vi "Navigation_start_cases.vi"() -> ()   [LabVIEW 2015]
uses:
  <vilib>/myRIO/Instrument Drivers/Onboard IO/PWM/typedefs/PWM Reference.ctl
  <vilib>/myRIO/Common/Instrument Driver Framework/Utilities/typedefs/myRIO Generic Hardware Reference.ctl
  <vilib>/myRIO/Common/Instrument Driver Framework/Utilities/typedefs/Hardware Version Enum.ctl
  <vilib>/myRIO/Common/Instrument Driver Framework/Utilities/typedefs/myRIO v1.0 Reference.ctl
  <vilib>/myRIO/Common/Instrument Driver Framework/Utilities/typedefs/Generic FPGA Reference.ctl
  <vilib>/myRIO/Common/Instrument Driver Framework/myRIO v1.0/PWM/typedefs/PWM Channels Enum.ctl
  <vilib>/myRIO/Instrument Drivers/Onboard IO/PWM/typedefs/PWM Configuration.ctl
  <vilib>/userdefined/High Color/nirio_resource_hc.ctl
  <vilib>/myRIO/Common/Instrument Driver Framework/myRIO v1.0/PWM/vis/myRIO v1.1 Open PWM.vi
  <vilib>/myRIO/Common/Instrument Driver Framework/Utilities/vis/Validate Channels.vi
  <vilib>/myRIO/Common/Instrument Driver Framework/myRIO v1.0/PWM/vis/myRIO v1.0 Reserve PWM.vi
  <vilib>/myRIO/Common/Instrument Driver Framework/myRIO v1.0/PWM/vis/myRIO v1.0 Build MUX Configuration PWM.vi
  <vilib>/myRIO/Common/Instrument Driver Framework/myRIO v1.0/Resource Manager/vis/myRIO v1.0 Reserve Channel List.vi
  <vilib>/myRIO/Common/Instrument Driver Framework/myRIO v1.0/Resource Manager/vis/myRIO v1.0 Create Configuration List.vi
  <vilib>/myRIO/Common/Instrument Driver Framework/myRIO v1.0/Resource Manager/vis/myRIO v1.0 Reserve Channel.vi
  <vilib>/myRIO/Common/Instrument Driver Framework/myRIO v1.0/Resource Manager/vis/myRIO v1.0 Unreserve Channel.vi
  <vilib>/myRIO/Common/Instrument Driver Framework/myRIO v1.0/Resource Manager/vis/myRIO v1.0 Build Mutex Name.vi
  <vilib>/FPGAPlugInAG/myRIO-1900/niLvFpga_Open_myRIO-1900.vi
  <vilib>/rvi/interface/common/dynamic/niFpgaDynamicAddResources.vi
  <vilib>/myRIO/Common/Instrument Driver Framework/Utilities/vis/FPGA Ref Manager.vi
  <vilib>/Utility/error.llb/Error Cluster From Error Code.vi
  <vilib>/myRIO/Common/Instrument Driver Framework/Utilities/vis/Ref Counter.vi
  <vilib>/rvi/errors/niLvFpgaAdjustHostInterfaceError.vi
  <vilib>/Utility/VariantDataType/GetNumericInfo.vi
  <vilib>/myRIO/Common/Instrument Driver Framework/myRIO v1.0/myRIO v1.1 Open.vi
  <vilib>/myRIO/Common/Instrument Driver Framework/Utilities/vis/IO Manager.vi
  <vilib>/myRIO/Common/Instrument Driver Framework/Utilities/vis/Configuration Manager.vi
  <vilib>/myRIO/Common/Instrument Driver Framework/myRIO v1.0/Resource Manager/vis/myRIO v1.0 Configure IO.vi
  <vilib>/myRIO/Common/Instrument Driver Framework/myRIO v1.0/myRIO v1.0 Close.vi
  <vilib>/myRIO/Common/Instrument Driver Framework/myRIO v1.0/PWM/vis/myRIO v1.0 Write PWM.vi
  <vilib>/addons/control/pid/pid.llb/PID (DBL).vi
  <vilib>/rvi/interface/nirviOpenFPGA/nirviOpenFPGA.xnode
  FPGA Bitfiles/NavigationProjec_FPGATarget2_FPGAMainNavigati_PWPHW8gwDxI.lvbitx
  <vilib>/rvi/interface/nirviReadWriteControl/nirviReadWriteControl.xnode
  <vilib>/myRIO/Instrument Drivers/Onboard IO/PWM/vis/myRIO PWM Open.xnode
  <vilib>/myRIO/Instrument Drivers/Onboard IO/PWM/PWM.lvlib
  <vilib>/myRIO/Instrument Drivers/Utilities/Utilities.lvlib
  NiFpgaLv.dll
  <vilib>/rvi/interface/Simulation/niFpgaSimulationCallBeginRW.vi
  <vilib>/addons/control/pid/NI_PID_pid.lvlib
panel:
  in  "t backward 6":u32=3000
  in  "Tab Control":enum32{"start a", "start b"}(tab)
  in  "?":T1(tab)=enum."back arc 4 4"
  in  "right 0":dbl=-0.05
  in  "left 0":dbl=-0.05
  in  "t backward 7":u32=3000
  in  "left 1":dbl=0.1
  in  "right 1":dbl=0.05
  in  "right 2":dbl=0.05
  in  "left 2":dbl=0.1
  in  "t backward":u32=3000
  in  "t forward":u32=750
  in  "t forward once":u32=3000
  in  "right once":dbl=0.05
  in  "left once":dbl=0.1
  in  "left 7":dbl=0.1
  in  "right 7":dbl=0.05
  in  "t forward 2":u32=750
  in  "left 6":dbl=0.1
  in  "right 6":dbl=0.05
  in  "t backward 2":u32=3000
  in  "left once 2":dbl=0.1
  in  "right once 2":dbl=0.05
  in  "t forward once 2":u32=3000
  in  "left 12":dbl=0.1
  in  "right 12":dbl=0.05
  in  "left 11":dbl=0.1
  in  "right 11":dbl=0.05
  in  "left 10":dbl=0.1
  in  "right 10":dbl=0.05
  in  "forward":u32=5000
  in  "timeforward":u32=750
  in  "timeback":u32=750
  in  "Tab Control 3":T2(tab)
  in  "left 15":dbl=-0.05
  in  "right 15":dbl=-0.05
  in  "t backward 8":u32=3000
  in  "left 5":dbl=0.1
  in  "right 5":dbl=0.05
  in  "left 4":dbl=0.1
  in  "right 4":dbl=0.05
  in  "left 3":dbl=0.1
  in  "right 3":dbl=0.05
  in  "forward 6":u32=750
  in  "backward 6":u32=750
  in  "onetime 6":u32=5000
  in  "t forward once 5":u32=3000
  in  "right once 5":dbl=0.05
  in  "left once 5":dbl=0.1
  in  "left 16":dbl=0.1
  in  "right 16":dbl=0.05
  in  "t backward 5":u32=3000
  in  "left 17":dbl=0.1
  in  "right 17":dbl=0.05
  in  "t forward 5":u32=750
  in  "start condition":dbl=4.0
  out "percent to goal":dbl
  out "x goal current":dbl=8.0
  out "big red button":i16
  out "y1ahead":dbl
  out "angle error":dbl
  out "y desired":dbl
  out "slope desired":dbl
  out "orientation theta desired":dbl
  out "current angle":dbl
  out "current y":dbl
  out "current x":dbl
  out "mining angle":dbl
  out "mining y":dbl
  out "mining x":dbl
  out "mining location":dbl=1.0
  out "distance to goal":dbl
  out "loc_y":dbl
  out "loc_x":dbl
  out "loc_theta":dbl
  in  "motor killswitch":bool=TRUE
  in  "set start position":bool
  in  "dumping complete":bool
  in  "digging complete?":bool
  in  "position good?":bool
  in  "state":dbl=5.0
  in  "x goal":dbl=8.0
  in  "Encoder Reset":bool
  out "scale":dbl=1.0
  out "reset x y 2":dbl
  out "stop motors":dbl
  out "encoder stop switch":dbl=1.0
  out "left wheels actual pwm":dbl
  out "right wheels actual pwm":dbl
  out "desired pwm right":dbl
  out "desired pwm left":dbl
  out "left setpoint":dbl
  out "right setpoint":dbl
  in  "PID Settings":enum32{"Right PID PWM", "Left PID PWM"}(tab)
  in  "output range right":cluster{"output high":dbl, "output low":dbl}={"output high"=0.13333, "output low"=-0.13333} {"output low" format="%.6f"; "output high" format="%.5f"}
  in  "PID gains right":T3={"proportional gain (Kc)"=0.002, "integral time (Ti, min)"=7e-07, "derivative time (Td, min)"=0.0} {"derivative time (Td, min)" format="%.8f"; "integral time (Ti, min)" format="%.8f"; "proportional gain (Kc)" format="%.8f"}
  out "dt out (s) right":dbl format="%.3f"
  out "PID feedback Right":dbl
  out "Elapsed Time (s) Right":dbl caption="Elapsed Time (s)"
  in  "pid reset right":bool
  in  "output range left":cluster{"output high":dbl, "output low":dbl}={"output high"=0.13333, "output low"=-0.13333} {"output low" format="%.6f"; "output high" format="%.5f"}
  in  "PID gains left":T3={"proportional gain (Kc)"=0.002, "integral time (Ti, min)"=7e-07, "derivative time (Td, min)"=0.0} {"derivative time (Td, min)" format="%.8f"; "integral time (Ti, min)" format="%.8f"; "proportional gain (Kc)" format="%.8f"}
  out "dt out (s) left":dbl format="%.3f"
  out "PID feedback Left":dbl
  out "Elapsed Time (s) Left":dbl caption="Elapsed Time (s)"
  in  "pid reset left":bool
  out "start angle":dbl=1.0
  out "start x":dbl=1.0
  out "start y":dbl
  in  "stuff that i dont want to mess with right now":T4(tab)
  out "RM Linear Velocity (rot/s)":dbl
  out "RR Rot Velocity (rot/s)":dbl
  out "LR Rot Velocity (rot/s)":dbl
  out "LM Rot Velocity (rot/s)":dbl
  out "LF Rot Velocity (rot/s)":dbl
  out "RF Linear Velocity (rot/s)":dbl
  out "Tick Count(mSec) 2":u32 caption="Tick Count(mSec)"
  out "y traveled 2":dbl
  out "x traveled 2":dbl
  out "y position 2":dbl
  out "x position 2":dbl
  out "y dot 2":dbl
  out "distance traveled 2":dbl
  out "psi dot 2":dbl
  out "x dot 2":dbl
  out ".not. x? 2":bool
  out ".not. x? 3":bool
  out "goal reached":bool=TRUE
  out "avg ENC.B":dbl
  out "avg ENC.A":dbl
  out "ENC.B_c.CNTR":i32
  out "ENC.B_b.CNTR":i32
  out "ENC.B_a.CNTR":i32
  out "ENC.A_c.CNTR":i32
  out "ENC.A_b.CNTR":i32
  out "ENC.A_a.CNTR":i32
  out "stage set point parameters":T5(tab)
  in  "x straight 1 end":dbl=2.0
  in  "ypstart straight 1":dbl
  in  "ystart":dbl=1.0
  in  "yend straight 1":dbl=2.0
  in  "ypend straight 1":dbl
  out "a":dbl
  out "b":dbl
  out "c":dbl
  out "d":dbl
  out "x turn end":dbl=7.0
  out "x straight 2 end":dbl=10.0
  in  "mining y 1":dbl=2.0
  in  "mining angle 1":dbl
  in  "mining x 1":dbl=-8.0
  in  "mining angle -1":dbl
  in  "mining y -1":dbl=4.0
  in  "mining x -1":dbl=-8.0
  out "left pwm":dbl(graph)
  out "right pwm":dbl(graph)
  out "SYS.SELECTA":u8 format="%08b"
  in  "R Min Linear Velocity (ft/s)":dbl=-2.0 format="%#_13g"
  in  "R Max Linear Velocity (ft/s)":dbl=2.0 format="%#_13g"
  in  "L Min Linear Velocity (ft/s)":dbl=-2.0 format="%#_13g"
  in  "L Max Linear Velocity (ft/s)":dbl=2.0 format="%#_13g"
  out "Current Rot Velocity (rot/s)":T6(graph)
  # "Position Information"
  # "straight arc back straight arc arc"
  # "same as the start a arc arc"
  # "move cases along"
  # "end state 0\ngo to state 1"
  # "end state 1\ngo to state 2"
  # "end state 2\ngo to state 3"
  # "end state 3\ngo to state 4"
  # "end state 4\ngo to state 0"
  # "same thing, redundant \nbut can be changed to \nsomething useful later"
  # "this must be true to \ninitialize the routine"
  # "go through the 3\n movement cases"
  # "go through the 3\n movement cases"
  # "Stop Flags \n1=go \n0=stop"
  # "PWM Setpoint"
  # "Initial condtions"
  # "Encoder Values"
  # "Motor Control Parameters"
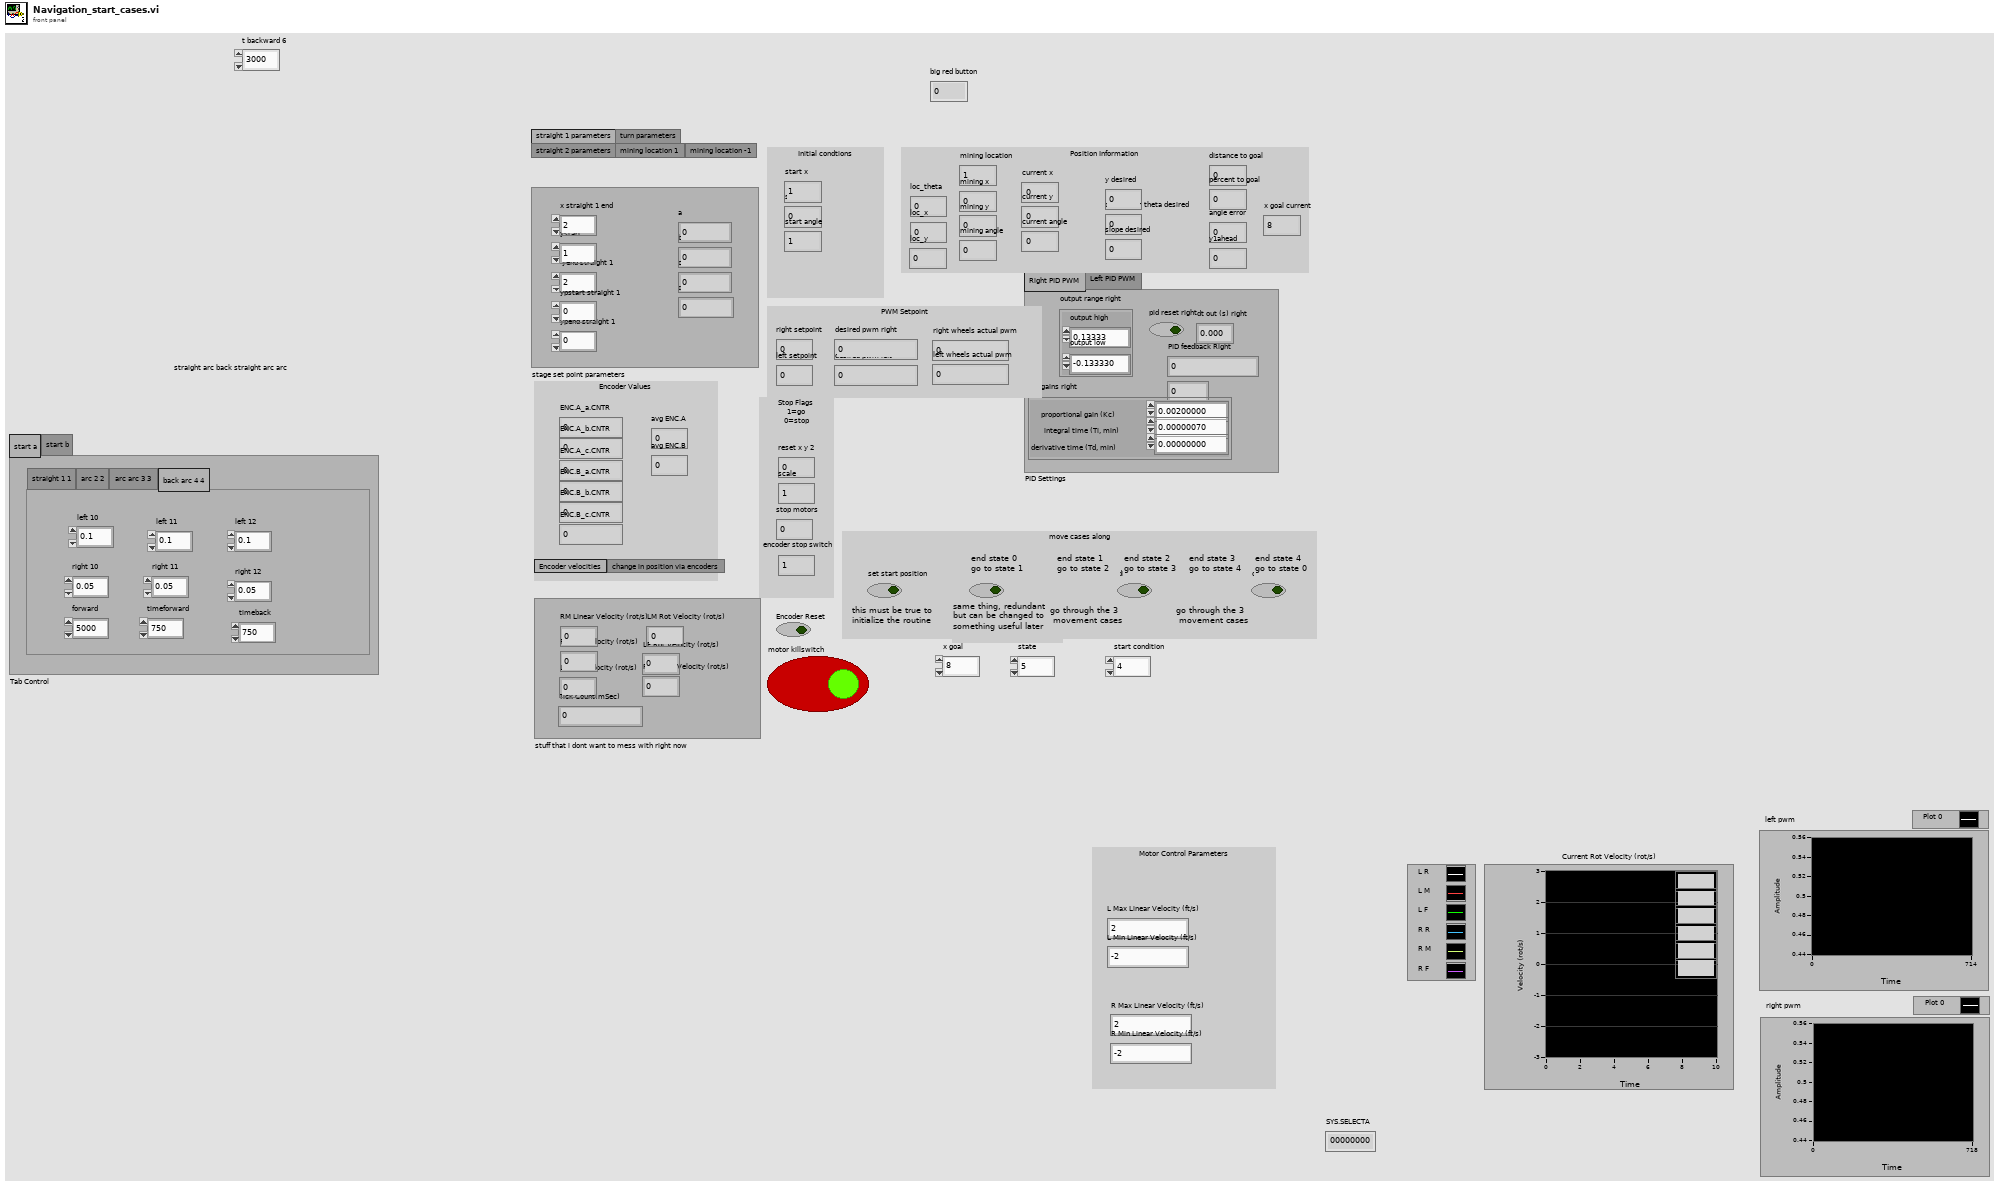
[diagram p1: front panel]
types:
  T1 = enum32{"straight 1 1", "arc 2 2", "arc arc 3 3 ", "back arc 4 4"}
  T2 = enum32{"straight 1 5", "arc 2 6", "arc arc 3", "back arc 4 7"}
  T3 = cluster{"proportional gain (Kc)":dbl, "integral time (Ti, min)":dbl, "derivative time (Td, min)":dbl}
  T4 = enum32{"Encoder velocities", "change in position via encoders"}
  T5 = enum32{"straight 1 parameters", "turn parameters", "straight 2 parameters", "mining location 1", "mining location -1"}
  T6 = cluster{"Rotational Velocity (RPS)":dbl, "Rotational Velocity (RPS)":dbl, "Rotational Velocity (RPS)":dbl, "Rotational Velocity (RPS)":dbl, "Rotational Velocity (RPS)":dbl, "Rotational Velocity (RPS)":dbl}
  T7 = typedef "nirio_resource_hc.ctl" = tag
  T8 = typedef "Hardware Version Enum.ctl" = enum16{"Unknown", "myRIO-1900", "myRIO-1950", "roboRIO"}
  T9 = typedef "PWM.lvlib/PWM Reference.ctl" = cluster{"myRIO Reference":T10, "PWM Channels Enum":T13, "PWM Configuration":T14}
  T10 = typedef "myRIO Generic Hardware Reference.ctl" = cluster{"myRIO Model":T8, "myRIO Hardware Reference":T11}
  T11 = typedef "myRIO v1.0 Reference.ctl" = cluster{"Generic FPGA Reference":T12, "Allow multiple opens":bool}
  T12 = typedef "Generic FPGA Reference.ctl" = refnum<k20>
  T13 = typedef "PWM Channels Enum.ctl" = enum16{"Not Connected", "C/PWM0", "C/PWM1", "A/PWM0", "A/PWM1", "A/PWM2", "B/PWM0", "B/PWM1", "B/PWM2", "PWM/PWM0", "PWM/PWM1", "PWM/PWM2", "PWM/PWM3", "PWM/PWM4", "PWM/PWM5", "PWM/PWM6", "PWM/PWM7", "PWM/PWM8", "PWM/PWM9"}
  T14 = typedef "PWM.lvlib/PWM Configuration.ctl" = cluster{"Frequency":dbl, "Duty Cycle":dbl}
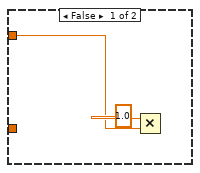
[diagram p3: hidden frame]
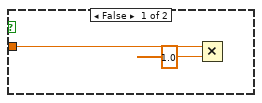
[diagram p4: hidden frame]
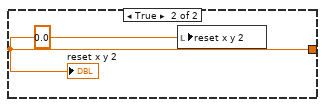
[diagram p5: hidden frame]
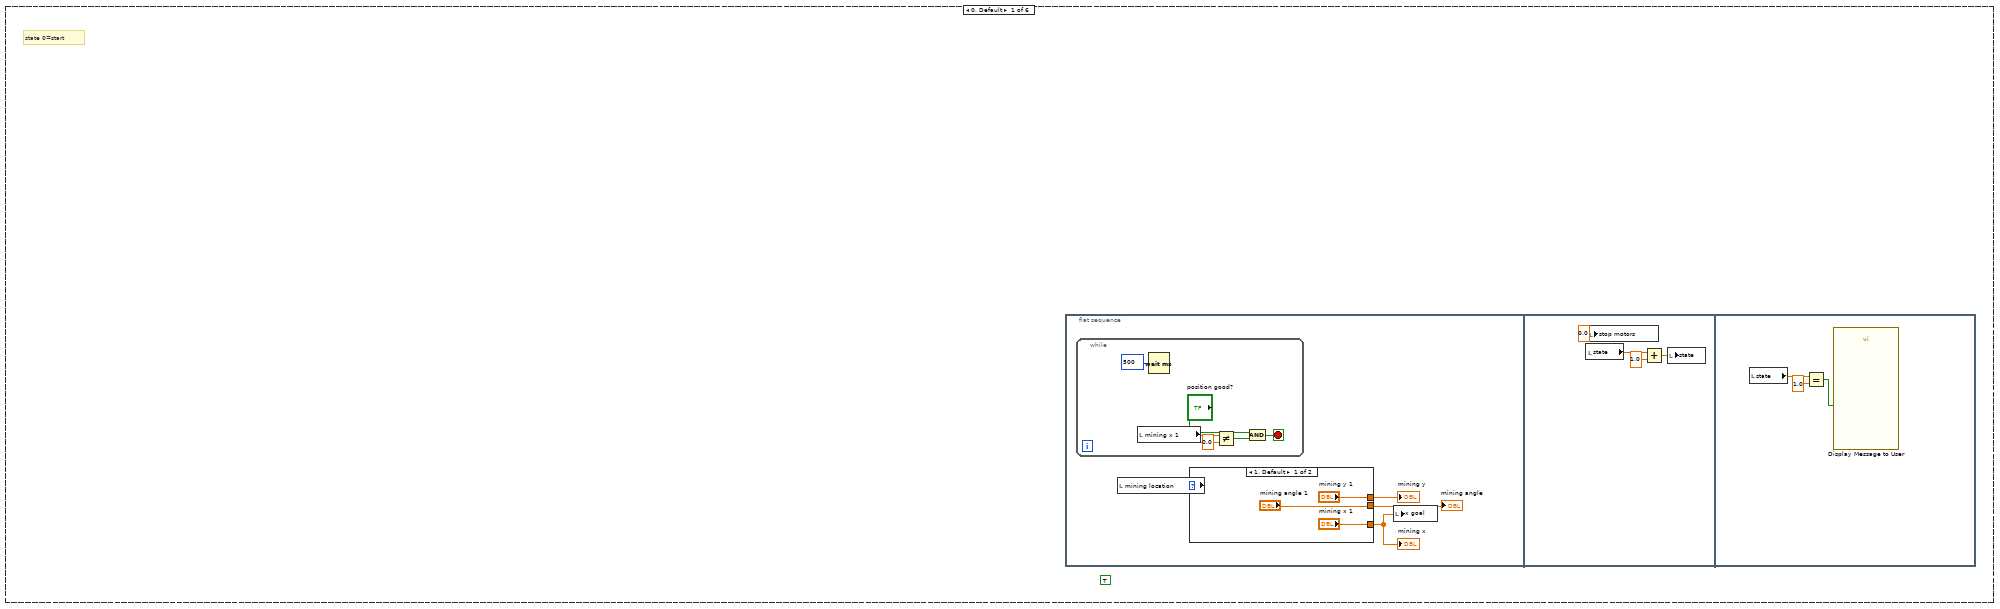
[diagram p6: hidden frame]
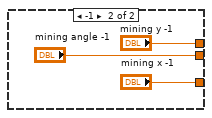
[diagram p7: hidden frame]
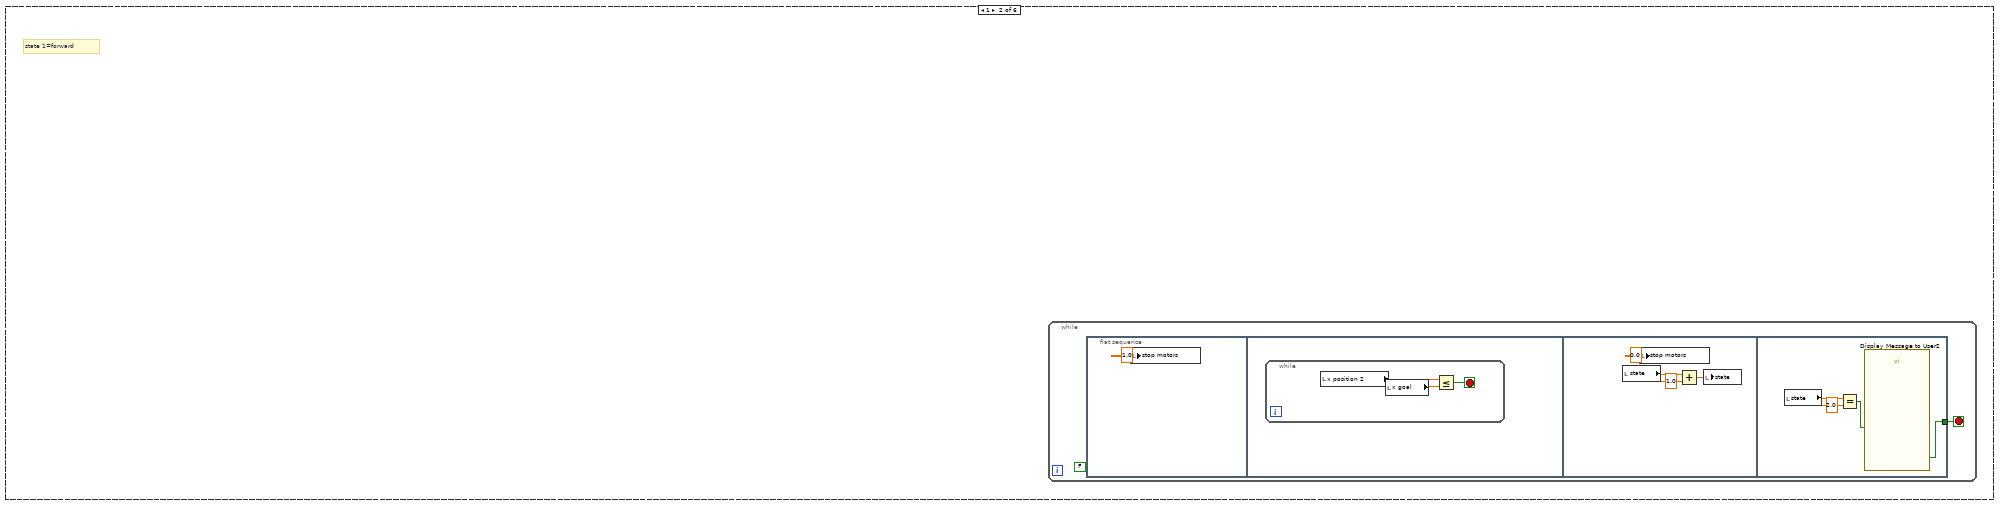
[diagram p8: hidden frame]
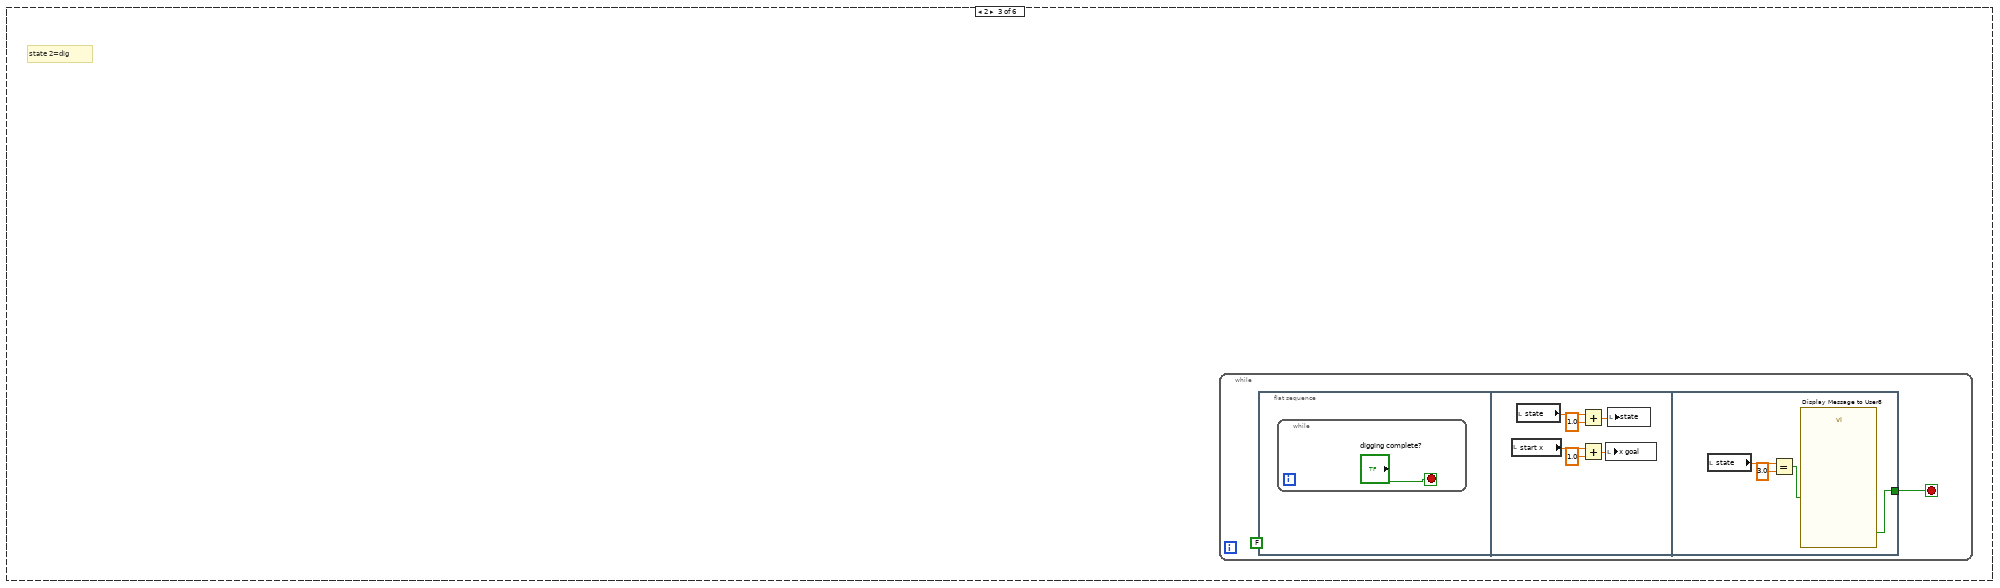
[diagram p9: hidden frame]
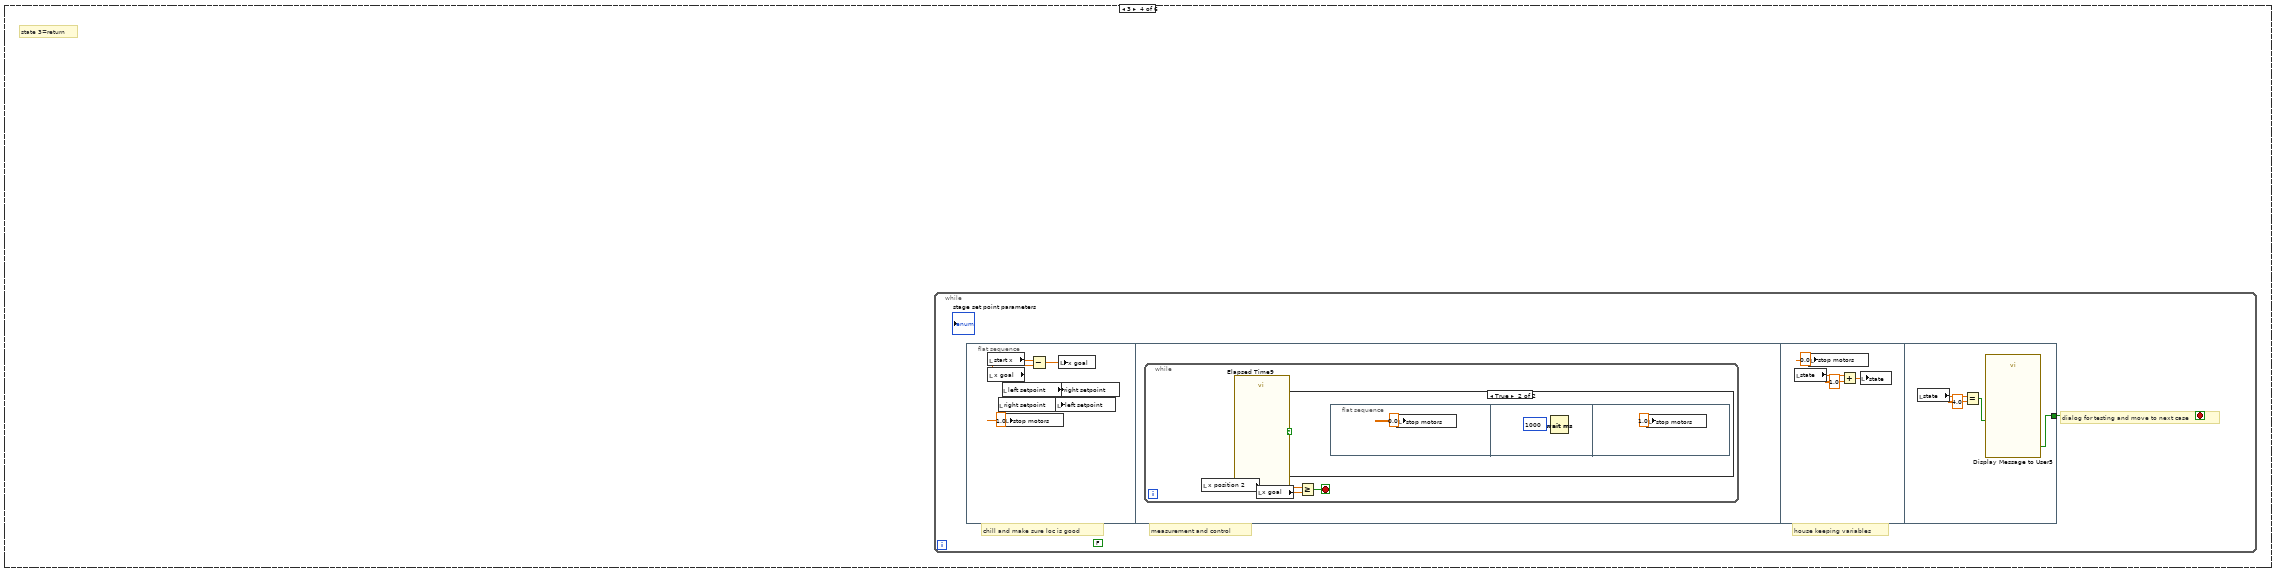
[diagram p10: hidden frame]
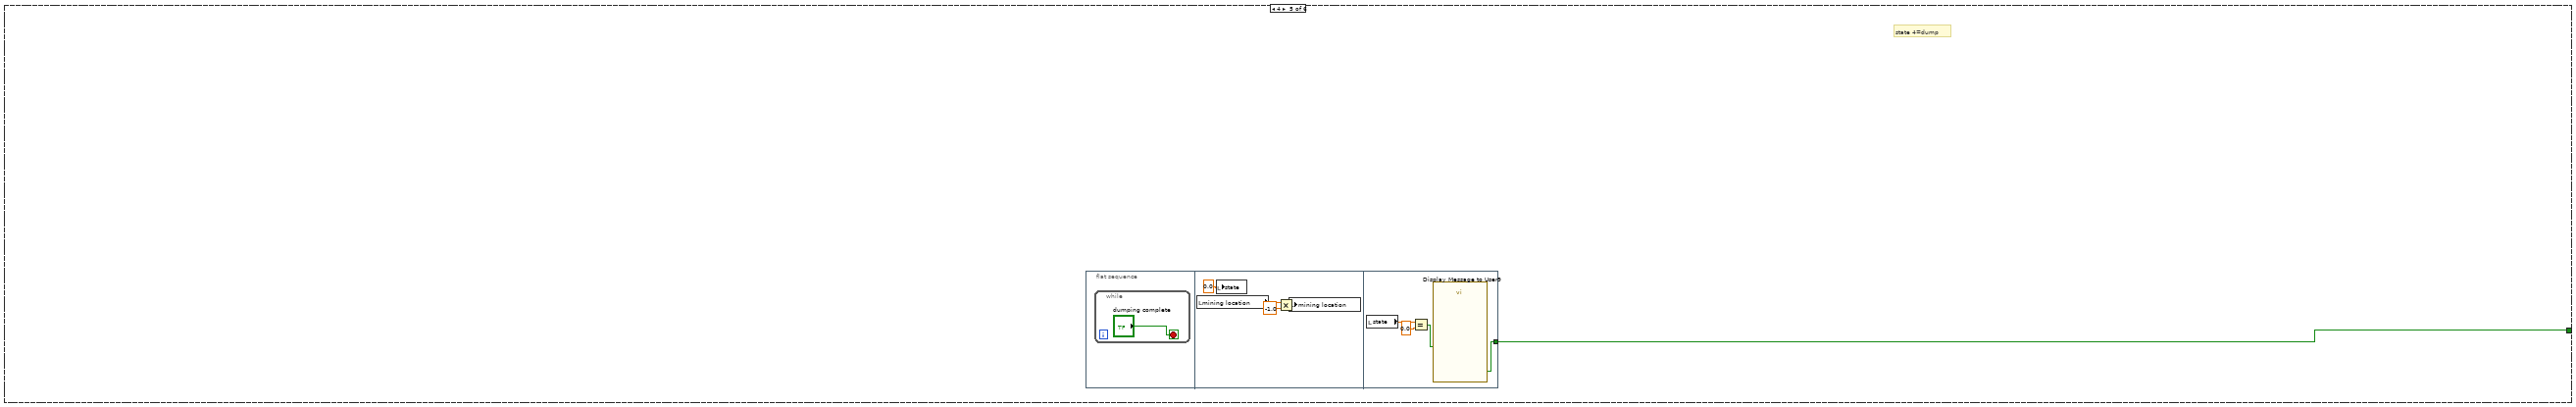
[diagram p12: hidden frame]
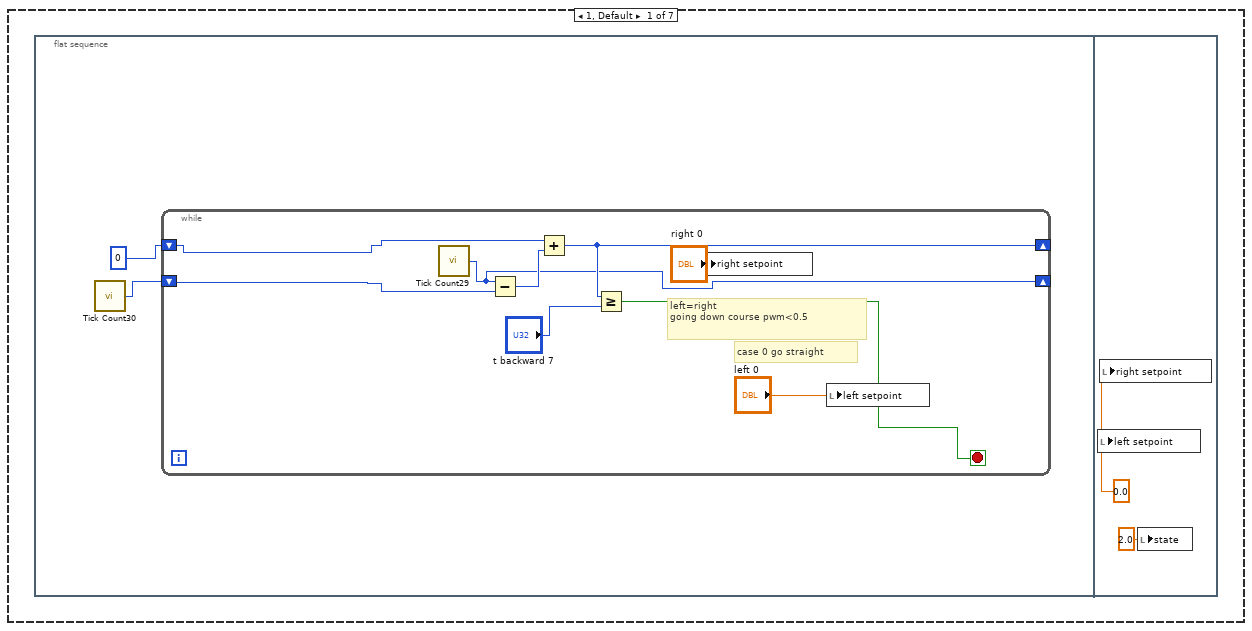
[diagram p13: hidden frame]
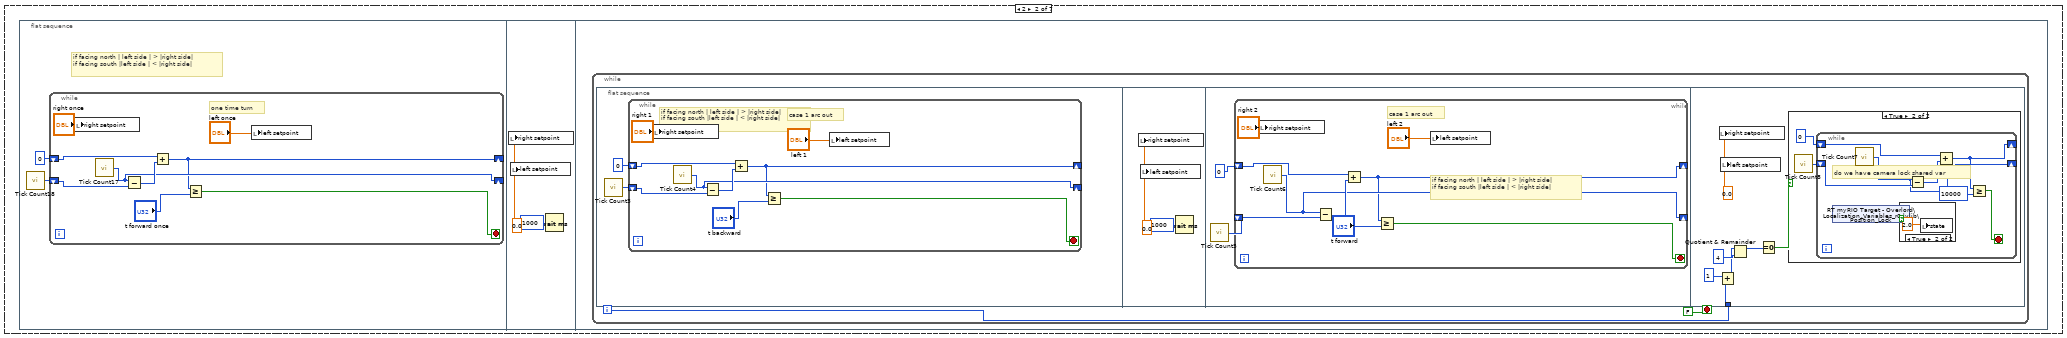
[diagram p14: hidden frame]
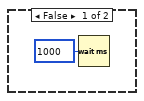
[diagram p15: hidden frame]
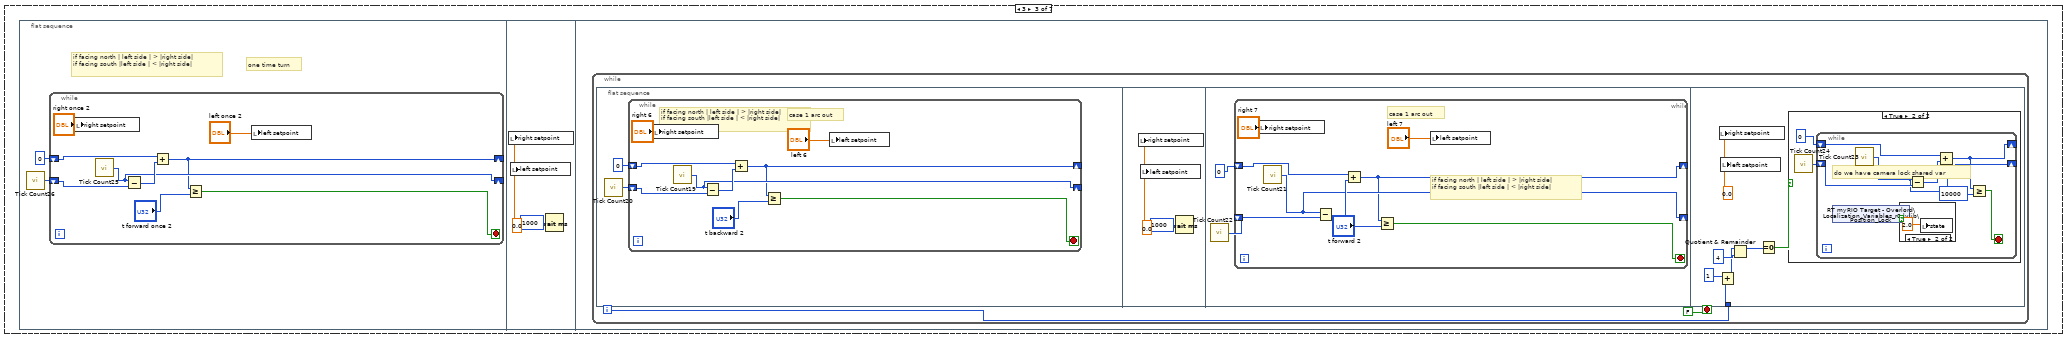
[diagram p17: hidden frame]
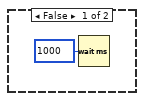
[diagram p18: hidden frame]
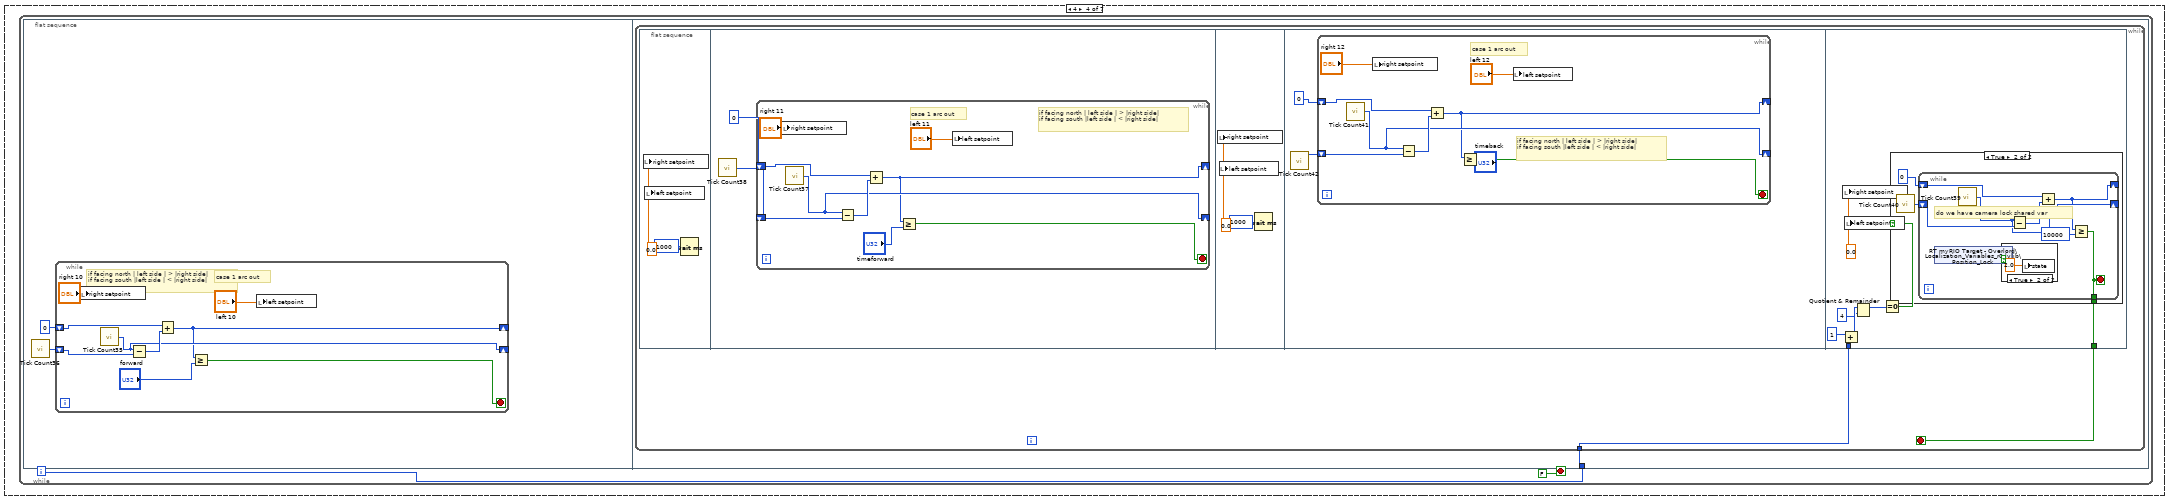
[diagram p20: hidden frame]
diagram:
  n1 = flat-sequence {
    tunnel: [w33] -> w30
    tunnel: [w33] -> w29
    tunnel: [w46] -> w28
    tunnel: [w61] -> w26
    tunnel: [w57] -> w24
    tunnel: [w56] -> w22
    tunnel: [w55] -> w20
    tunnel: [w54] -> w18
    tunnel: [w53] -> w16
    tunnel: ["L Max Linear Velocity (ft/s)"] -> w14
    tunnel: ["L Min Linear Velocity (ft/s)"] -> w12
    tunnel: ["R Max Linear Velocity (ft/s)"] -> w10
    tunnel: ["R Min Linear Velocity (ft/s)"] -> w8
    tunnel: [w48] -> w6
    tunnel: w30 -> [w47]
    tunnel: [w47] -> w4
    tunnel: w29 -> [w48]
    tunnel: [w46] -> w2
    tunnel: w28 -> [w187]
    tunnel: [w187] -> w27
    tunnel: w26 -> [w186]
    tunnel: [w186] -> w25
    tunnel: w24 -> [w185]
    tunnel: [w185] -> w23
    tunnel: w22 -> [w184]
    tunnel: [w184] -> w21
    tunnel: w20 -> [w183]
    tunnel: [w183] -> w19
    tunnel: w18 -> [w182]
    tunnel: [w182] -> w17
    tunnel: w16 -> [w181]
    tunnel: [w181] -> w15
    tunnel: w14 -> [w180]
    tunnel: [w180] -> w13
    tunnel: w12 -> [w179]
    tunnel: [w179] -> w11
    tunnel: w10 -> [w178]
    tunnel: [w178] -> w9
    tunnel: w8 -> [w177]
    tunnel: [w177] -> w7
    tunnel: w6 -> [w176]
    tunnel: [w176] -> w5
    tunnel: w4 -> [w175]
    tunnel: [w175] -> w3
    tunnel: w2 -> [w174]
    tunnel: [w174] -> w1
    tunnel: w27 -> [_]
    tunnel: w25 -> [w198]
    tunnel: w23 -> [w204]
    tunnel: w21 -> [w201]
    tunnel: w19 -> [w200]
    tunnel: w17 -> [w199]
    tunnel: w15 -> [w203]
    tunnel: w13 -> [_]
    tunnel: w11 -> [_]
    tunnel: w9 -> [_]
    tunnel: w7 -> [_]
    tunnel: w5 -> [w206]
    tunnel: w3 -> [w205]
    tunnel: w1 -> [w202]
    frame #0 {
      n2 = xnode "Open FPGA VI Reference"("resource name"=tag "RIO0") -> ("FPGA VI Reference Out"=w32:refnum<k20>)  [unwired: 1 in, 1 out]
      n3 = call <vilib>:"Set Custom Bitfile.vi"("Custom FPGA Reference In"=w32) -> ("Custom FPGA Reference Out"=w34:refnum<k20>)  [unwired: 9 in, 1 out]
      n4 = flat-sequence {
        tunnel: w34 -> [w39]
        tunnel: [w37] -> w36
        tunnel: w36 -> [w41]
        tunnel: [w41] -> w35
        tunnel: w35 -> [w44]
        tunnel: [w43] -> w33
        frame #0 {
          w38 = u8 32 ("SYS.SELECTA")
          w40 = u8 3 ("ENC.B_c.CNFG")
          n5 = xnode "Read/Write Control"("FPGA VI Reference In"=w39, "ENC.A_a.CNFG"=w40, "ENC.A_b.CNFG"=w40, "ENC.A_c.CNFG"=w40, "ENC.B_a.CNFG"=w40, "ENC.B_b.CNFG"=w40, "ENC.B_c.CNFG"=w40, "SYS.SELECTA"=w38, "SYS.SELECTB"=w38) -> ("FPGA VI Reference Out"=w37:refnum<k20>)  [unwired: 1 in, 1 out]
        }
        frame #1 {
          n6 = Wait (ms)(milliseconds to wait=u32 10) -> ()  [unwired: 1 out]
        }
        frame #2 {
          w45 = u8 1 ("ENC.B_c.CNFG")
          n7 = xnode "Read/Write Control"("FPGA VI Reference In"=w44, "ENC.A_a.CNFG"=w45, "ENC.A_b.CNFG"=w45, "ENC.A_c.CNFG"=w45, "ENC.B_a.CNFG"=w45, "ENC.B_b.CNFG"=w45, "ENC.B_c.CNFG"=w45) -> ("FPGA VI Reference Out"=w43:refnum<k20>)  [unwired: 1 in, 1 out]
        }
      }
    }
    frame #1 {
      w58 = 0.5 ("Duty Cycle")
      w46 = 333.333 ("Frequency [Hz]")
      w72 = tag "B/PWM2"  # Right rear ch
      w73 = tag "B/PWM0"  # Right mid ch
      w74 = tag "B/PWM1"  # Right front ch
      w75 = tag "A/PWM2"  # Left rear ch
      w76 = tag "A/PWM1"  # Left mid ch
      w77 = tag "A/PWM0"  # Left front ch
      n8 = xnode "Right  Front"("Channel Name"=w74) -> ("PWM Ref Out"=w68:T9)  [unwired: 2 in, 1 out]
      n9 = xnode "Right  Rear"("Channel Name"=w72) -> ("PWM Ref Out"=w66:T9)  [unwired: 2 in, 1 out]
      n10 = xnode "Left Front"("Channel Name"=w77) -> ("PWM Ref Out"=w71:T9)  [unwired: 2 in, 1 out]
      n11 = xnode "Right  Mid"("Channel Name"=w73) -> ("PWM Ref Out"=w67:T9)  [unwired: 2 in, 1 out]
      n12 = xnode "Left Rear"("Channel Name"=w75) -> ("PWM Ref Out"=w69:T9)  [unwired: 2 in, 1 out]
      n13 = xnode "Left Mid"("Channel Name"=w76) -> ("PWM Ref Out"=w70:T9)  [unwired: 2 in, 1 out]
      n14 = call <vilib>:"Set Frequency.vi"("Frequency [Hz]"=w46, "PWM Ref In"=w71) -> ("PWM Ref Out"=w65:T9)  [unwired: 7 in, 1 out]
      n15 = call <vilib>:"Set Frequency.vi"("Frequency [Hz]"=w46, "PWM Ref In"=w69) -> ("PWM Ref Out"=w60:T9)  [unwired: 7 in, 1 out]
      n16 = call <vilib>:"Set Frequency.vi"("Frequency [Hz]"=w46, "PWM Ref In"=w70) -> ("PWM Ref Out"=w59:T9)  [unwired: 7 in, 1 out]
      n17 = call <vilib>:"Set Frequency.vi"("Frequency [Hz]"=w46, "PWM Ref In"=w67) -> ("PWM Ref Out"=w63:T9)  [unwired: 7 in, 1 out]
      n18 = call <vilib>:"Set Frequency.vi"("Frequency [Hz]"=w46, "PWM Ref In"=w68) -> ("PWM Ref Out"=w62:T9)  [unwired: 7 in, 1 out]
      n19 = call <vilib>:"Set Frequency.vi"("Frequency [Hz]"=w46, "PWM Ref In"=w66) -> ("PWM Ref Out"=w64:T9)  [unwired: 7 in, 1 out]
      n20 = call <vilib>:"Set Duty Cycle.vi"("Duty Cycle"=w58, "PWM Ref In"=w65) -> ("PWM Ref Out"=w53:T9)  [unwired: 7 in, 1 out]
      n21 = call <vilib>:"Set Duty Cycle.vi"("Duty Cycle"=w58, "PWM Ref In"=w60) -> ("PWM Ref Out"=w61:T9)  [unwired: 7 in, 1 out]
      n22 = call <vilib>:"Set Duty Cycle.vi"("Duty Cycle"=w58, "PWM Ref In"=w59) -> ("PWM Ref Out"=w54:T9)  [unwired: 7 in, 1 out]
      n23 = call <vilib>:"Set Duty Cycle.vi"("Duty Cycle"=w58, "PWM Ref In"=w63) -> ("PWM Ref Out"=w56:T9)  [unwired: 7 in, 1 out]
      n24 = call <vilib>:"Set Duty Cycle.vi"("Duty Cycle"=w58, "PWM Ref In"=w62) -> ("PWM Ref Out"=w57:T9)  [unwired: 7 in, 1 out]
      n25 = call <vilib>:"Set Duty Cycle.vi"("Duty Cycle"=w58, "PWM Ref In"=w64) -> ("PWM Ref Out"=w55:T9)  [unwired: 7 in, 1 out]
    }
    frame #2 {
      n26 = while {
        stop <- w188 stop-if-true
        n27 = case shown="True" "set start position" {
          selector: "set start position" -> [_ w195]
          tunnel: [_ w195] -> w188
          frame False {
          }
          frame True {
            n28 = shared-variable "RT myRIO Target - Overlord\\Localization_Variables_r0.lvlib\\loc_y"() -> (→"start y":dbl)  [unwired: 1 in, 1 out]
            n29 = shared-variable "RT myRIO Target - Overlord\\Localization_Variables_r0.lvlib\\loc_x"() -> (→"start x":dbl)  [unwired: 1 in, 1 out]
            n30 = shared-variable "RT myRIO Target - Overlord\\Localization_Variables_r0.lvlib\\loc_theta"() -> (→"start angle":dbl)  [unwired: 1 in, 1 out]
            n31 = Wait (ms)(milliseconds to wait=u32 500) -> ()  [unwired: 1 out]
            "stop motors" <- 1.0 ("stop motors")
          }
        }
      }
    }
    frame #3 {
      (unwired) FALSE
      # "Uses quadrature encoder tick count to calculate rotational and linear velocity for a wheel."
      # "20ms loop delay to allow the encoder to travel far enough for a good update. 20ms provides 50Hz update rate to match motor PWM output rate."
      n32 = while {
        stop <- w265 stop-if-true
        n33 = case shown="5" "state" {
          tunnel: [_ _ _ _ w336 _] -> w265
          frame 0, Default {
            (unwired) TRUE
            # "state 0=start"
            n34 = flat-sequence {
              frame #0 {
                n35 = while {
                  stop <- w276 stop-if-true
                  n36 = local read "mining x 1"() -> (w281:dbl)
                  n37 = Wait (ms)(milliseconds to wait=u32 500) -> ()  [unwired: 1 out]
                  n38 = Not Equal?(x=w281, y=0.0) -> (x != y?=w277:bool)
                  n39 = And(x="position good?", y=w277) -> (x .and. y?=w276:bool)
                }
                n40 = local read "mining location"() -> (w269:dbl)
                n41 = case shown="1, Default" w269 {
                  tunnel: ["mining x 1" "mining x -1"] -> w266
                  tunnel: ["mining y 1" "mining y -1"] -> w268
                  tunnel: ["mining angle 1" "mining angle -1"] -> w267
                  frame 1, Default {
                  }
                  frame -1 {
                  }
                }
                "mining x" <- w266
                "mining y" <- w268
                "mining angle" <- w267
                n42 = local write "x goal"(w266) -> ()
              }
              frame #1 {
                n43 = local read "state"() -> (w283:dbl)
                n44 = local write "stop motors"(0.0 ("stop motors")) -> ()
                n45 = Add(x=w283, y=1.0) -> (x+y=w285:dbl)
                n46 = local write "state"(w285) -> ()
              }
              frame #2 {
                n47 = local read "state"() -> (w288:dbl)
                n48 = Equal?(x=w288, y=1.0) -> (x = y?=w286:bool)
                n49 = call "Display Message to User"("Enable"=w286) -> ()  [unwired: 9 in, 2 out]
              }
            }
          }
          frame 1 {
            # "state 1=forward"
            n50 = while {
              stop <- w289 stop-if-true
              (unwired) FALSE
              n51 = flat-sequence {
                tunnel: [w298] -> w289
                frame #0 {
                  n52 = local write "stop motors"(1.0) -> ()
                }
                frame #1 {
                  n53 = while {
                    stop <- w293 stop-if-true
                    n54 = local read "x position 2"() -> (w291:dbl)
                    n55 = local read "x goal"() -> (w292:dbl)
                    n56 = Less Or Equal?(x=w291, y=w292) -> (x <= y?=w293:bool)
                  }
                }
                frame #2 {
                  n57 = local read "state"() -> (w294:dbl)
                  n58 = local write "stop motors"(0.0) -> ()
                  n59 = Add(x=w294, y=1.0) -> (x+y=w296:dbl)
                  n60 = local write "state"(w296) -> ()
                }
                frame #3 {
                  n61 = local read "state"() -> (w301:dbl)
                  n62 = Equal?(x=w301, y=2.0) -> (x = y?=w299:bool)
                  n63 = call "Display Message to User2"("Enable"=w299) -> ("OK"=w298:bool)  [unwired: 9 in, 1 out]
                }
              }
            }
          }
          frame 2 {
            # "state 2=dig"
            n64 = while {
              stop <- w302 stop-if-true
              (unwired) FALSE
              n65 = flat-sequence {
                tunnel: [w310] -> w302
                frame #0 {
                  n66 = while {
                    stop <- "digging complete?" stop-if-true
                  }
                }
                frame #1 {
                  n67 = local read "start x"() -> (w306:dbl)
                  n68 = local read "state"() -> (w308:dbl)
                  n69 = Add(x=w308, y=1.0) -> (x+y=w307:dbl)
                  n70 = Add(x=w306, y=1.0) -> (x+y=w305:dbl)
                  n71 = local write "x goal"(w305) -> ()
                  n72 = local write "state"(w307) -> ()
                }
                frame #2 {
                  n73 = local read "state"() -> (w313:dbl)
                  n74 = Equal?(x=w313, y=3.0) -> (x = y?=w311:bool)
                  n75 = call "Display Message to User8"("Enable"=w311) -> ("OK"=w310:bool)  [unwired: 9 in, 1 out]
                }
              }
            }
          }
          frame 3 {
            # "state 3=return"
            n76 = while {
              stop <- w314 stop-if-true
              (unwired) FALSE
              # "dialog for testing and move to next case"
              # "measurement and control"
              # "chill and make sure loc is good"
              # "house keeping variables"
              n77 = flat-sequence {
                tunnel: [w332] -> w314
                frame #0 {
                  n78 = local read "start x"() -> (w317:dbl)
                  n79 = local read "x goal"() -> (w315:dbl)
                  n80 = local read "right setpoint"() -> (w318:dbl)
                  n81 = local read "left setpoint"() -> (w319:dbl)
                  n82 = local write "stop motors"(1.0) -> ()
                  n83 = Subtract(x=w317, y=w315) -> (x-y=w316:dbl)
                  n84 = local write "right setpoint"(w319) -> ()
                  n85 = local write "left setpoint"(w318) -> ()
                  n86 = local write "x goal"(w316) -> ()
                }
                frame #1 {
                  n87 = while {
                    stop <- w324 stop-if-true
                    n88 = local read "x position 2"() -> (w321:dbl)
                    n89 = call "Elapsed Time9"() -> ("Time has Elapsed"=w323:bool)  [unwired: 12 in, 7 out]
                    n90 = local read "x goal"() -> (w322:dbl)
                    n91 = case shown="True" w323 {
                      frame False {
                      }
                      frame True {
                        n92 = flat-sequence {
                          frame #0 {
                            n93 = local write "stop motors"(0.0) -> ()
                          }
                          frame #1 {
                            n94 = Wait (ms)(milliseconds to wait=u32 1000) -> ()  [unwired: 1 out]
                          }
                          frame #2 {
                            n95 = local write "stop motors"(1.0) -> ()
                          }
                        }
                      }
                    }
                    n96 = Greater Or Equal?(x=w321, y=w322) -> (x >= y?=w324:bool)
                  }
                }
                frame #2 {
                  n97 = local read "state"() -> (w329:dbl)
                  n98 = local write "stop motors"(0.0) -> ()
                  n99 = Add(x=w329, y=1.0) -> (x+y=w331:dbl)
                  n100 = local write "state"(w331) -> ()
                }
                frame #3 {
                  n101 = local read "state"() -> (w335:dbl)
                  n102 = Equal?(x=w335, y=4.0) -> (x = y?=w333:bool)
                  n103 = call "Display Message to User5"("Enable"=w333) -> ("OK"=w332:bool)  [unwired: 9 in, 1 out]
                }
              }
            }
          }
          frame 4 {
            # "state 4=dump"
            n104 = flat-sequence {
              tunnel: [w342] -> w336
              frame #0 {
                n105 = while {
                  stop <- "dumping complete" stop-if-true
                }
              }
              frame #1 {
                n106 = local read "mining location"() -> (w340:dbl)
                n107 = local write "state"(0.0) -> ()
                n108 = Multiply(x=w340, y=-1.0) -> (x*y=w338:dbl)
                n109 = local write "mining location"(w338) -> ()
              }
              frame #2 {
                n110 = local read "state"() -> (w345:dbl)
                n111 = Equal?(x=w345, y=0.0) -> (x = y?=w343:bool)
                n112 = call "Display Message to User9"("Enable"=w343) -> ("OK"=w342:bool)  [unwired: 9 in, 1 out]
              }
            }
          }
          frame 5 {
            n113 = case shown="6" "start condition" {
              frame 1, Default {
                n114 = flat-sequence {
                  frame #0 {
                    n115 = call "Tick Count30"() -> ("Tick Count(mSec)"=w347:u32)
                    n116 = while {
                      shift-right: [w350] -> _
                      shift-left: w347 -> [w351]
                      shift-right: [w353] -> _
                      shift-left: 0 -> [w349]
                      stop <- w352 stop-if-true
                      # "left=right\ngoing down course pwm<0.5"
                      # "case 0 go straight"
                      n117 = call "Tick Count29"() -> ("Tick Count(mSec)"=w350:u32)
                      n118 = Subtract(x=w350, y=w351) -> (x-y=w354:u32)
                      n119 = Add(x=w349, y=w354) -> (x+y=w353:u32)
                      n120 = Greater Or Equal?(x=w353, y="t backward 7") -> (x >= y?=w352:bool)
                      n121 = local write "right setpoint"("right 0") -> ()
                      n122 = local write "left setpoint"("left 0") -> ()
                    }
                  }
                  frame #1 {
                    w359 = 0.0
                    n123 = local write "left setpoint"(w359) -> ()
                    n124 = local write "right setpoint"(w359) -> ()
                    n125 = local write "state"(2.0 ("state")) -> ()
                  }
                }
              }
              frame 2 {
                n126 = flat-sequence {
                  frame #0 {
                    # "if facing north | left side | > |right side|\nif facing south |left side | < |right side|"
                    n127 = call "Tick Count18"() -> ("Tick Count(mSec)"=w361:u32)
                    n128 = while {
                      shift-right: [w364] -> _
                      shift-left: 0 -> [w366]
                      shift-right: [w365] -> _
                      shift-left: w361 -> [w368]
                      stop <- w363 stop-if-true
                      # "one time turn"
                      n129 = local write "right setpoint"("right once") -> ()
                      n130 = call "Tick Count17"() -> ("Tick Count(mSec)"=w365:u32)
                      n131 = Subtract(x=w365, y=w368) -> (x-y=w367:u32)
                      n132 = Add(x=w366, y=w367) -> (x+y=w364:u32)
                      n133 = Greater Or Equal?(x=w364, y="t forward once") -> (x >= y?=w363:bool)
                      n134 = local write "left setpoint"("left once") -> ()
                    }
                  }
                  frame #1 {
                    w371 = 0.0
                    n135 = local write "right setpoint"(w371) -> ()
                    n136 = local write "left setpoint"(w371) -> ()
                    n137 = Wait (ms)(milliseconds to wait=u32 1000) -> ()  [unwired: 1 out]
                  }
                  frame #2 {
                    n138 = while {
                      i -> [w373]
                      stop <- FALSE stop-if-true
                      n139 = flat-sequence {
                        tunnel: w373 -> [w405]
                        frame #0 {
                          n140 = call "Tick Count3"() -> ("Tick Count(mSec)"=w375:u32)
                          n141 = while {
                            shift-right: [w379] -> _
                            shift-left: 0 -> [w381]
                            shift-right: [w380] -> _
                            shift-left: w375 -> [w383]
                            stop <- w378 stop-if-true
                            # "if facing north | left side | > |right side|\nif facing south |left side | < |right side|"
                            # "case 1 arc out"
                            n142 = local write "right setpoint"("right 1") -> ()
                            n143 = call "Tick Count4"() -> ("Tick Count(mSec)"=w380:u32)
                            n144 = Subtract(x=w380, y=w383) -> (x-y=w382:u32)
                            n145 = Add(x=w381, y=w382) -> (x+y=w379:u32)
                            n146 = Greater Or Equal?(x=w379, y="t backward") -> (x >= y?=w378:bool)
                            n147 = local write "left setpoint"("left 1") -> ()
                          }
                        }
                        frame #1 {
                          w387 = 0.0
                          n148 = local write "right setpoint"(w387) -> ()
                          n149 = local write "left setpoint"(w387) -> ()
                          n150 = Wait (ms)(milliseconds to wait=u32 1000) -> ()  [unwired: 1 out]
                        }
                        frame #2 {
                          n151 = call "Tick Count5"() -> ("Tick Count(mSec)"=w389:u32)
                          n152 = while {
                            shift-right: [w392] -> _
                            shift-left: 0 -> [w395]
                            shift-right: [w393] -> _
                            shift-left: w389 -> [w396]
                            stop <- w391 stop-if-true
                            # "if facing north | left side | > |right side|\nif facing south |left side | < |right side|"
                            # "case 1 arc out"
                            n153 = local write "right setpoint"("right 2") -> ()
                            n154 = call "Tick Count6"() -> ("Tick Count(mSec)"=w393:u32)
                            n155 = Subtract(x=w393, y=w396) -> (x-y=w394:u32)
                            n156 = Add(x=w395, y=w394) -> (x+y=w392:u32)
                            n157 = Greater Or Equal?(x=w392, y="t forward") -> (x >= y?=w391:bool)
                            n158 = local write "left setpoint"("left 2") -> ()
                          }
                        }
                        frame #3 {
                          w404 = 0.0
                          n159 = Add(x=1, y=w405) -> (x+y=w400:i32)
                          n160 = local write "right setpoint"(w404) -> ()
                          n161 = local write "left setpoint"(w404) -> ()
                          n162 = Quotient & Remainder(x=w400, y=4) -> (x-y*floor(x/y)=w402:i32)  [unwired: 1 out]
                          n163 = Equal To 0?(x=w402) -> (x = 0?=w401:bool)
                          n164 = case shown="True" w401 {
                            frame False {
                              n165 = Wait (ms)(milliseconds to wait=u32 1000) -> ()  [unwired: 1 out]
                            }
                            frame True {
                              n166 = call "Tick Count8"() -> ("Tick Count(mSec)"=w407:u32)
                              n167 = while {
                                shift-right: [w410] -> _
                                shift-left: 0 -> [w413]
                                shift-right: [w411] -> _
                                shift-left: w407 -> [w412]
                                stop <- w409 stop-if-true
                                # "do we have camera lock shared var"
                                n168 = shared-variable "RT myRIO Target - Overlord\\Localization_Variables_r0.lvlib\\Position_Lock"() -> (w416:bool)  [unwired: 1 in, 1 out]
                                n169 = call "Tick Count7"() -> ("Tick Count(mSec)"=w411:u32)
                                n170 = case shown="True" w416 {
                                frame False {
                                }
                                frame True {
                                n171 = local write "state"(2.0) -> ()
                                }
                                }
                                n172 = Subtract(x=w411, y=w412) -> (x-y=w415:u32)
                                n173 = Add(x=w413, y=w415) -> (x+y=w410:u32)
                                n174 = Greater Or Equal?(x=w410, y=u32 10000) -> (x >= y?=w409:bool)
                              }
                            }
                          }
                        }
                      }
                    }
                  }
                }
              }
              frame 3 {
                n175 = flat-sequence {
                  frame #0 {
                    # "one time turn"
                    # "if facing north | left side | > |right side|\nif facing south |left side | < |right side|"
                    n176 = call "Tick Count26"() -> ("Tick Count(mSec)"=w419:u32)
                    n177 = while {
                      shift-right: [w422] -> _
                      shift-left: 0 -> [w424]
                      shift-right: [w423] -> _
                      shift-left: w419 -> [w426]
                      stop <- w421 stop-if-true
                      n178 = local write "right setpoint"("right once 2") -> ()
                      n179 = call "Tick Count25"() -> ("Tick Count(mSec)"=w423:u32)
                      n180 = Subtract(x=w423, y=w426) -> (x-y=w425:u32)
                      n181 = Add(x=w424, y=w425) -> (x+y=w422:u32)
                      n182 = Greater Or Equal?(x=w422, y="t forward once 2") -> (x >= y?=w421:bool)
                      n183 = local write "left setpoint"("left once 2") -> ()
                    }
                  }
                  frame #1 {
                    w429 = 0.0
                    n184 = local write "right setpoint"(w429) -> ()
                    n185 = local write "left setpoint"(w429) -> ()
                    n186 = Wait (ms)(milliseconds to wait=u32 1000) -> ()  [unwired: 1 out]
                  }
                  frame #2 {
                    n187 = while {
                      i -> [w431]
                      stop <- FALSE stop-if-true
                      n188 = flat-sequence {
                        tunnel: w431 -> [w463]
                        frame #0 {
                          n189 = call "Tick Count20"() -> ("Tick Count(mSec)"=w433:u32)
                          n190 = while {
                            shift-right: [w437] -> _
                            shift-left: 0 -> [w439]
                            shift-right: [w438] -> _
                            shift-left: w433 -> [w441]
                            stop <- w436 stop-if-true
                            # "if facing north | left side | > |right side|\nif facing south |left side | < |right side|"
                            # "case 1 arc out"
                            n191 = local write "right setpoint"("right 6") -> ()
                            n192 = call "Tick Count19"() -> ("Tick Count(mSec)"=w438:u32)
                            n193 = Subtract(x=w438, y=w441) -> (x-y=w440:u32)
                            n194 = Add(x=w439, y=w440) -> (x+y=w437:u32)
                            n195 = Greater Or Equal?(x=w437, y="t backward 2") -> (x >= y?=w436:bool)
                            n196 = local write "left setpoint"("left 6") -> ()
                          }
                        }
                        frame #1 {
                          w445 = 0.0
                          n197 = local write "right setpoint"(w445) -> ()
                          n198 = local write "left setpoint"(w445) -> ()
                          n199 = Wait (ms)(milliseconds to wait=u32 1000) -> ()  [unwired: 1 out]
                        }
                        frame #2 {
                          n200 = call "Tick Count22"() -> ("Tick Count(mSec)"=w447:u32)
                          n201 = while {
                            shift-right: [w450] -> _
                            shift-left: 0 -> [w453]
                            shift-right: [w451] -> _
                            shift-left: w447 -> [w454]
                            stop <- w449 stop-if-true
                            # "if facing north | left side | > |right side|\nif facing south |left side | < |right side|"
                            # "case 1 arc out"
                            n202 = local write "right setpoint"("right 7") -> ()
                            n203 = call "Tick Count21"() -> ("Tick Count(mSec)"=w451:u32)
                            n204 = Subtract(x=w451, y=w454) -> (x-y=w452:u32)
                            n205 = Add(x=w453, y=w452) -> (x+y=w450:u32)
                            n206 = Greater Or Equal?(x=w450, y="t forward 2") -> (x >= y?=w449:bool)
                            n207 = local write "left setpoint"("left 7") -> ()
                          }
                        }
                        frame #3 {
                          w462 = 0.0
                          n208 = Add(x=1, y=w463) -> (x+y=w458:i32)
                          n209 = local write "right setpoint"(w462) -> ()
                          n210 = local write "left setpoint"(w462) -> ()
                          n211 = Quotient & Remainder(x=w458, y=4) -> (x-y*floor(x/y)=w460:i32)  [unwired: 1 out]
                          n212 = Equal To 0?(x=w460) -> (x = 0?=w459:bool)
                          n213 = case shown="True" w459 {
                            frame False {
                              n214 = Wait (ms)(milliseconds to wait=u32 1000) -> ()  [unwired: 1 out]
                            }
                            frame True {
                              n215 = call "Tick Count24"() -> ("Tick Count(mSec)"=w465:u32)
                              n216 = while {
                                shift-right: [w468] -> _
                                shift-left: 0 -> [w471]
                                shift-right: [w469] -> _
                                shift-left: w465 -> [w470]
                                stop <- w467 stop-if-true
                                # "do we have camera lock shared var"
                                n217 = shared-variable "RT myRIO Target - Overlord\\Localization_Variables_r0.lvlib\\Position_Lock"() -> (w474:bool)  [unwired: 1 in, 1 out]
                                n218 = call "Tick Count23"() -> ("Tick Count(mSec)"=w469:u32)
                                n219 = case shown="True" w474 {
                                frame False {
                                }
                                frame True {
                                n220 = local write "state"(2.0) -> ()
                                }
                                }
                                n221 = Subtract(x=w469, y=w470) -> (x-y=w473:u32)
                                n222 = Add(x=w471, y=w473) -> (x+y=w468:u32)
                                n223 = Greater Or Equal?(x=w468, y=u32 10000) -> (x >= y?=w467:bool)
                              }
                            }
                          }
                        }
                      }
                    }
                  }
                }
              }
              frame 4 {
                n224 = while {
                  i -> [w476]
                  stop <- FALSE stop-if-true
                  n225 = flat-sequence {
                    tunnel: w476 -> [w489]
                    frame #0 {
                      n226 = call "Tick Count36"() -> ("Tick Count(mSec)"=w478:u32)
                      n227 = while {
                        shift-right: [w482] -> _
                        shift-left: 0 -> [w484]
                        shift-right: [w483] -> _
                        shift-left: w478 -> [w486]
                        stop <- w481 stop-if-true
                        # "if facing north | left side | > |right side|\nif facing south |left side | < |right side|"
                        # "case 1 arc out"
                        n228 = local write "right setpoint"("right 10") -> ()
                        n229 = call "Tick Count35"() -> ("Tick Count(mSec)"=w483:u32)
                        n230 = Subtract(x=w483, y=w486) -> (x-y=w485:u32)
                        n231 = Add(x=w484, y=w485) -> (x+y=w482:u32)
                        n232 = Greater Or Equal?(x=w482, y="forward") -> (x >= y?=w481:bool)
                        n233 = local write "left setpoint"("left 10") -> ()
                      }
                    }
                    frame #1 {
                      n234 = while {
                        tunnel: w489 -> [w491]
                        stop <- w490 stop-if-true
                        n235 = flat-sequence {
                          tunnel: w491 -> [w519]
                          tunnel: [w518] -> w490
                          frame #0 {
                            w492 = 0.0
                            n236 = local write "right setpoint"(w492) -> ()
                            n237 = local write "left setpoint"(w492) -> ()
                            n238 = Wait (ms)(milliseconds to wait=u32 1000) -> ()  [unwired: 1 out]
                          }
                          frame #1 {
                            n239 = call "Tick Count38"() -> ("Tick Count(mSec)"=w494:u32)
                            n240 = while {
                              shift-right: [w497] -> _
                              shift-left: 0 -> [w500]
                              shift-right: [w498] -> _
                              shift-left: w494 -> [w501]
                              stop <- w496 stop-if-true
                              # "if facing north | left side | > |right side|\nif facing south |left side | < |right side|"
                              # "case 1 arc out"
                              n241 = local write "right setpoint"("right 11") -> ()
                              n242 = call "Tick Count37"() -> ("Tick Count(mSec)"=w498:u32)
                              n243 = Subtract(x=w498, y=w501) -> (x-y=w499:u32)
                              n244 = Add(x=w500, y=w499) -> (x+y=w497:u32)
                              n245 = Greater Or Equal?(x=w497, y="timeforward") -> (x >= y?=w496:bool)
                              n246 = local write "left setpoint"("left 11") -> ()
                            }
                          }
                          frame #2 {
                            w505 = 0.0
                            n247 = local write "right setpoint"(w505) -> ()
                            n248 = local write "left setpoint"(w505) -> ()
                            n249 = Wait (ms)(milliseconds to wait=u32 1000) -> ()  [unwired: 1 out]
                          }
                          frame #3 {
                            n250 = call "Tick Count42"() -> ("Tick Count(mSec)"=w507:u32)
                            n251 = while {
                              shift-right: [w510] -> _
                              shift-left: 0 -> [w513]
                              shift-right: [w511] -> _
                              shift-left: w507 -> [w514]
                              stop <- w509 stop-if-true
                              # "if facing north | left side | > |right side|\nif facing south |left side | < |right side|"
                              # "case 1 arc out"
                              n252 = call "Tick Count41"() -> ("Tick Count(mSec)"=w511:u32)
                              n253 = local write "right setpoint"("right 12") -> ()
                              n254 = Subtract(x=w511, y=w514) -> (x-y=w512:u32)
                              n255 = Add(x=w513, y=w512) -> (x+y=w510:u32)
                              n256 = Greater Or Equal?(x=w510, y="timeback") -> (x >= y?=w509:bool)
                              n257 = local write "left setpoint"("left 12") -> ()
                            }
                          }
                          frame #4 {
                            w520 = 0.0
                            n258 = Add(x=1, y=w519) -> (x+y=w524:i32)
                            n259 = local write "right setpoint"(w520) -> ()
                            n260 = local write "left setpoint"(w520) -> ()
                            n261 = Quotient & Remainder(x=w524, y=4) -> (x-y*floor(x/y)=w522:i32)  [unwired: 1 out]
                            n262 = Equal To 0?(x=w522) -> (x = 0?=w523:bool)
                            n263 = case shown="True" w523 {
                              tunnel: [_ w527] -> w518
                              frame False {
                                n264 = Wait (ms)(milliseconds to wait=u32 1000) -> ()  [unwired: 1 out]
                              }
                              frame True {
                                n265 = call "Tick Count40"() -> ("Tick Count(mSec)"=w528:u32)
                                n266 = while {
                                shift-right: [w531] -> _
                                shift-left: 0 -> [w534]
                                shift-right: [w532] -> _
                                shift-left: w528 -> [w533]
                                tunnel: [w530] -> w527
                                stop <- w530 stop-if-true
                                # "do we have camera lock shared var"
                                n267 = shared-variable "RT myRIO Target - Overlord\\Localization_Variables_r0.lvlib\\Position_Lock"() -> (w537:bool)  [unwired: 1 in, 1 out]
                                n268 = call "Tick Count39"() -> ("Tick Count(mSec)"=w532:u32)
                                n269 = case shown="True" w537 {
                                frame False {
                                }
                                frame True {
                                n270 = local write "state"(2.0) -> ()
                                }
                                }
                                n271 = Subtract(x=w532, y=w533) -> (x-y=w536:u32)
                                n272 = Add(x=w534, y=w536) -> (x+y=w531:u32)
                                n273 = Greater Or Equal?(x=w531, y=u32 10000) -> (x >= y?=w530:bool)
                                }
                              }
                            }
                          }
                        }
                      }
                    }
                  }
                }
              }
              frame 5 {
                n274 = flat-sequence {
                  frame #0 {
                    n275 = while {
                      shift-right: [w543] -> _
                      shift-left: _ -> [w539]
                      shift-right: [w542] -> _
                      shift-left: _ -> [w540]
                      stop <- w541 stop-if-true
                      # "left=right\ngoing down course pwm<0.5"
                      # "case 0 go straight"
                      n276 = local write "right setpoint"("right 15") -> ()
                      n277 = local write "left setpoint"("left 15") -> ()
                      n278 = call "Tick Count31"() -> ("Tick Count(mSec)"=w542:u32)
                      n279 = Subtract(x=w542, y=w540) -> (x-y=w544:u32)
                      n280 = Add(x=w539, y=w544) -> (x+y=w543:u32)
                      n281 = Greater Or Equal?(x=w543, y="t backward 8") -> (x >= y?=w541:bool)
                    }
                  }
                  frame #1 {
                    w549 = 0.0
                    n282 = local write "left setpoint"(w549) -> ()
                    n283 = local write "right setpoint"(w549) -> ()
                    n284 = local write "state"(2.0 ("state")) -> ()
                  }
                }
              }
              frame 6 {
                n285 = while {
                  i -> [w550]
                  stop <- FALSE stop-if-true
                  n286 = flat-sequence {
                    tunnel: w550 -> [w563]
                    frame #0 {
                      # "back up straight"
                      n287 = call "Tick Count10"() -> ("Tick Count(mSec)"=w552:u32)
                      n288 = while {
                        shift-right: [w556] -> _
                        shift-left: 0 -> [w558]
                        shift-right: [w557] -> _
                        shift-left: w552 -> [w560]
                        stop <- w554 stop-if-true
                        # "if facing north | left side | > |right side|\nif facing south |left side | < |right side|"
                        # "case 1 arc out"
                        n289 = local write "right setpoint"("right 3") -> ()
                        n290 = call "Tick Count9"() -> ("Tick Count(mSec)"=w557:u32)
                        n291 = Subtract(x=w557, y=w560) -> (x-y=w559:u32)
                        n292 = Add(x=w558, y=w559) -> (x+y=w556:u32)
                        n293 = Greater Or Equal?(x=w556, y="onetime 6") -> (x >= y?=w554:bool)
                        n294 = local write "left setpoint"("left 3") -> ()
                      }
                    }
                    frame #1 {
                      n295 = while {
                        tunnel: w563 -> [w565]
                        stop <- w564 stop-if-true
                        n296 = flat-sequence {
                          tunnel: w565 -> [w593]
                          tunnel: [w592] -> w564
                          frame #0 {
                            w566 = 0.0
                            n297 = local write "right setpoint"(w566) -> ()
                            n298 = local write "left setpoint"(w566) -> ()
                            n299 = Wait (ms)(milliseconds to wait=u32 1000) -> ()  [unwired: 1 out]
                          }
                          frame #1 {
                            n300 = call "Tick Count12"() -> ("Tick Count(mSec)"=w568:u32)
                            n301 = while {
                              shift-right: [w571] -> _
                              shift-left: 0 -> [w574]
                              shift-right: [w572] -> _
                              shift-left: w568 -> [w575]
                              stop <- w570 stop-if-true
                              # "if facing north | left side | > |right side|\nif facing south |left side | < |right side|"
                              # "case 1 arc out"
                              n302 = local write "right setpoint"("right 4") -> ()
                              n303 = call "Tick Count11"() -> ("Tick Count(mSec)"=w572:u32)
                              n304 = Subtract(x=w572, y=w575) -> (x-y=w573:u32)
                              n305 = Add(x=w574, y=w573) -> (x+y=w571:u32)
                              n306 = Greater Or Equal?(x=w571, y="backward 6") -> (x >= y?=w570:bool)
                              n307 = local write "left setpoint"("left 4") -> ()
                            }
                          }
                          frame #2 {
                            w579 = 0.0
                            n308 = local write "right setpoint"(w579) -> ()
                            n309 = local write "left setpoint"(w579) -> ()
                            n310 = Wait (ms)(milliseconds to wait=u32 1000) -> ()  [unwired: 1 out]
                          }
                          frame #3 {
                            n311 = call "Tick Count16"() -> ("Tick Count(mSec)"=w581:u32)
                            n312 = while {
                              shift-right: [w584] -> _
                              shift-left: 0 -> [w587]
                              shift-right: [w585] -> _
                              shift-left: w581 -> [w588]
                              stop <- w583 stop-if-true
                              # "if facing north | left side | > |right side|\nif facing south |left side | < |right side|"
                              # "case 1 arc out"
                              n313 = call "Tick Count15"() -> ("Tick Count(mSec)"=w585:u32)
                              n314 = local write "right setpoint"("right 5") -> ()
                              n315 = Subtract(x=w585, y=w588) -> (x-y=w586:u32)
                              n316 = Add(x=w587, y=w586) -> (x+y=w584:u32)
                              n317 = Greater Or Equal?(x=w584, y="forward 6") -> (x >= y?=w583:bool)
                              n318 = local write "left setpoint"("left 5") -> ()
                            }
                          }
                          frame #4 {
                            w594 = 0.0
                            n319 = Add(x=1, y=w593) -> (x+y=w598:i32)
                            n320 = local write "right setpoint"(w594) -> ()
                            n321 = local write "left setpoint"(w594) -> ()
                            n322 = Quotient & Remainder(x=w598, y=4) -> (x-y*floor(x/y)=w596:i32)  [unwired: 1 out]
                            n323 = Equal To 0?(x=w596) -> (x = 0?=w597:bool)
                            n324 = case shown="True" w597 {
                              tunnel: [_ w601] -> w592
                              frame False {
                                n325 = Wait (ms)(milliseconds to wait=u32 1000) -> ()  [unwired: 1 out]
                              }
                              frame True {
                                n326 = call "Tick Count14"() -> ("Tick Count(mSec)"=w602:u32)
                                n327 = while {
                                shift-right: [w605] -> _
                                shift-left: 0 -> [w608]
                                shift-right: [w606] -> _
                                shift-left: w602 -> [w607]
                                tunnel: [w604] -> w601
                                stop <- w604 stop-if-true
                                # "do we have camera lock shared var"
                                n328 = shared-variable "RT myRIO Target - Overlord\\Localization_Variables_r0.lvlib\\Position_Lock"() -> (w611:bool)  [unwired: 1 in, 1 out]
                                n329 = call "Tick Count13"() -> ("Tick Count(mSec)"=w606:u32)
                                n330 = case shown="True" w611 {
                                frame False {
                                }
                                frame True {
                                n331 = local write "state"(2.0) -> ()
                                }
                                }
                                n332 = Subtract(x=w606, y=w607) -> (x-y=w610:u32)
                                n333 = Add(x=w608, y=w610) -> (x+y=w605:u32)
                                n334 = Greater Or Equal?(x=w605, y=u32 10000) -> (x >= y?=w604:bool)
                                }
                              }
                            }
                          }
                        }
                      }
                    }
                  }
                }
              }
              frame 7 {
                n335 = flat-sequence {
                  frame #0 {
                    # "if facing north | left side | > |right side|\nif facing south |left side | < |right side|"
                    n336 = call "Tick Count50"() -> ("Tick Count(mSec)"=w614:u32)
                    n337 = while {
                      shift-right: [w617] -> _
                      shift-left: 0 -> [w619]
                      shift-right: [w618] -> _
                      shift-left: w614 -> [w621]
                      stop <- w616 stop-if-true
                      # "one time turn"
                      n338 = local write "right setpoint"("right once 5") -> ()
                      n339 = call "Tick Count49"() -> ("Tick Count(mSec)"=w618:u32)
                      n340 = Subtract(x=w618, y=w621) -> (x-y=w620:u32)
                      n341 = Add(x=w619, y=w620) -> (x+y=w617:u32)
                      n342 = Greater Or Equal?(x=w617, y="t forward once 5") -> (x >= y?=w616:bool)
                      n343 = local write "left setpoint"("left once 5") -> ()
                    }
                  }
                  frame #1 {
                    w624 = 0.0
                    n344 = local write "right setpoint"(w624) -> ()
                    n345 = local write "left setpoint"(w624) -> ()
                    n346 = Wait (ms)(milliseconds to wait=u32 1000) -> ()  [unwired: 1 out]
                  }
                  frame #2 {
                    n347 = while {
                      i -> [w626]
                      stop <- FALSE stop-if-true
                      n348 = flat-sequence {
                        tunnel: w626 -> [w658]
                        frame #0 {
                          n349 = call "Tick Count44"() -> ("Tick Count(mSec)"=w628:u32)
                          n350 = while {
                            shift-right: [w632] -> _
                            shift-left: 0 -> [w634]
                            shift-right: [w633] -> _
                            shift-left: w628 -> [w636]
                            stop <- w631 stop-if-true
                            # "if facing north | left side | > |right side|\nif facing south |left side | < |right side|"
                            # "case 1 arc out"
                            n351 = local write "right setpoint"("right 16") -> ()
                            n352 = call "Tick Count43"() -> ("Tick Count(mSec)"=w633:u32)
                            n353 = Subtract(x=w633, y=w636) -> (x-y=w635:u32)
                            n354 = Add(x=w634, y=w635) -> (x+y=w632:u32)
                            n355 = Greater Or Equal?(x=w632, y="t backward 5") -> (x >= y?=w631:bool)
                            n356 = local write "left setpoint"("left 16") -> ()
                          }
                        }
                        frame #1 {
                          w640 = 0.0
                          n357 = local write "right setpoint"(w640) -> ()
                          n358 = local write "left setpoint"(w640) -> ()
                          n359 = Wait (ms)(milliseconds to wait=u32 1000) -> ()  [unwired: 1 out]
                        }
                        frame #2 {
                          n360 = call "Tick Count46"() -> ("Tick Count(mSec)"=w642:u32)
                          n361 = while {
                            shift-right: [w645] -> _
                            shift-left: 0 -> [w648]
                            shift-right: [w646] -> _
                            shift-left: w642 -> [w649]
                            stop <- w644 stop-if-true
                            # "if facing north | left side | > |right side|\nif facing south |left side | < |right side|"
                            # "case 1 arc out"
                            n362 = local write "right setpoint"("right 17") -> ()
                            n363 = call "Tick Count45"() -> ("Tick Count(mSec)"=w646:u32)
                            n364 = Subtract(x=w646, y=w649) -> (x-y=w647:u32)
                            n365 = Add(x=w648, y=w647) -> (x+y=w645:u32)
                            n366 = Greater Or Equal?(x=w645, y="t forward 5") -> (x >= y?=w644:bool)
                            n367 = local write "left setpoint"("left 17") -> ()
                          }
                        }
                        frame #3 {
                          w657 = 0.0
                          n368 = Add(x=1, y=w658) -> (x+y=w653:i32)
                          n369 = local write "right setpoint"(w657) -> ()
                          n370 = local write "left setpoint"(w657) -> ()
                          n371 = Quotient & Remainder(x=w653, y=4) -> (x-y*floor(x/y)=w655:i32)  [unwired: 1 out]
                          n372 = Equal To 0?(x=w655) -> (x = 0?=w654:bool)
                          n373 = case shown="True" w654 {
                            frame False {
                              n374 = Wait (ms)(milliseconds to wait=u32 1000) -> ()  [unwired: 1 out]
                            }
                            frame True {
                              n375 = call "Tick Count48"() -> ("Tick Count(mSec)"=w660:u32)
                              n376 = while {
                                shift-right: [w663] -> _
                                shift-left: 0 -> [w666]
                                shift-right: [w664] -> _
                                shift-left: w660 -> [w665]
                                stop <- w662 stop-if-true
                                # "do we have camera lock shared var"
                                n377 = shared-variable "RT myRIO Target - Overlord\\Localization_Variables_r0.lvlib\\Position_Lock"() -> (w669:bool)  [unwired: 1 in, 1 out]
                                n378 = call "Tick Count47"() -> ("Tick Count(mSec)"=w664:u32)
                                n379 = case shown="True" w669 {
                                frame False {
                                }
                                frame True {
                                n380 = local write "state"(2.0) -> ()
                                }
                                }
                                n381 = Subtract(x=w664, y=w665) -> (x-y=w668:u32)
                                n382 = Add(x=w666, y=w668) -> (x+y=w663:u32)
                                n383 = Greater Or Equal?(x=w663, y=u32 10000) -> (x >= y?=w662:bool)
                              }
                            }
                          }
                        }
                      }
                    }
                  }
                }
              }
            }
          }
        }
      }
      n384 = call "Tick Count"() -> ("Tick Count(uSec)"=w207:u32)
      n385 = call "Tick Count28"() -> ("Tick Count(mSec)"=w197:u32)
      n386 = while {
        shift-right: [w210] -> _
        shift-left: 0 -> [w212]
        shift-right: [w211] -> _
        shift-left: w197 -> [w214]
        stop <- w209 stop-if-true
        n387 = call "Tick Count27"() -> ("Tick Count(mSec)"=w211:u32)
        n388 = Subtract(x=w211, y=w214) -> (x-y=w213:u32)
        n389 = Add(x=w212, y=w213) -> (x+y=w210:u32)
        n390 = Greater Or Equal?(x=w210, y="t backward 6") -> (x >= y?=w209:bool)
      }
      n391 = while {
        stop <- FALSE stop-if-true
        n392 = shared-variable "RT myRIO Target - Overlord\\Localization_Variables_r0.lvlib\\loc_y"() -> (→"loc_y":dbl)  [unwired: 1 in, 1 out]
        n393 = shared-variable "RT myRIO Target - Overlord\\Localization_Variables_r0.lvlib\\loc_x"() -> (→"loc_x":dbl)  [unwired: 1 in, 1 out]
        n394 = local read "x position 2"() -> (w671:dbl)
        n395 = shared-variable "RT myRIO Target - Overlord\\Localization_Variables_r0.lvlib\\loc_theta"() -> (→"loc_theta":dbl)  [unwired: 1 in, 1 out]
        n396 = local read "x goal"() -> (w674:dbl)
        "x goal current" <- w674
        n397 = Subtract(x=w671, y=w674) -> (x-y=→"distance to goal":dbl)
      }
      n398 = flat-sequence {
        frame #0 {
          # "this calculates from the \nmeasured start to the desired end"
          n399 = local read "x straight 1 end"() -> (w254:dbl)
          n400 = local read "start x"() -> (w255:dbl)
          n401 = call "path coefs.vi"("ypend"="ypend straight 1", "ypstart"="ypstart straight 1", "yend"="yend straight 1", "ystart"="ystart", "xend"=w254, "xstart"=w255) -> ("d"=→"d":dbl, "c"=→"c":dbl, "b"=→"b":dbl, "a"=→"a":dbl)  [unwired: 2 in]
        }
      }
      n402 = while {
        stop <- FALSE stop-if-true
        n403 = local read "current x"() -> (w248:dbl)
        n404 = local read "a"() -> (w252:dbl)
        n405 = local read "b"() -> (w251:dbl)
        n406 = local read "d"() -> (w249:dbl)
        n407 = local read "c"() -> (w250:dbl)
        n408 = formula code="yshould=(a*x**3)/3+(b*x**2)/3+(c*x)/3+d/3;\ny1ahead=(a*(x+1)**3)/3+(b*(x+1)**2)/3+(c*(x+1))/3+d/3;\nslope=(a*x**2 + (2*b*x)/3 + c/3);\nrobot_orientation_theta=(atan(slope));\nleftwheel_x=(-1*sin(robot_orientation_theta)+x);\nrightwheel_x=(1*sin(robot_orientation_theta)+x);\nleftwheel_y=(1*cos(robot_orientation_theta)+yshould);\nrightwheel_y=(-1*cos(robot_orientation_theta)+yshould);"("a"=w252, "b"=w251, "c"=w250, "d"=w249, "x"=w248) -> ("yshould"=→"y desired":dbl, "slope"=→"slope desired":dbl, "robot_orientation_theta"=w245:dbl, "y1ahead"=→"y1ahead":dbl)  [unwired: 4 out]
        "orientation theta desired" <- w245
        n409 = local read "current angle"() -> (w244:dbl)
        n410 = Subtract(x=w245, y=w244) -> (x-y=→"angle error":dbl)
      }
      n411 = while {
        tunnel: w203 -> [w708]
        tunnel: [w709] -> _
        tunnel: w202 -> [w696]
        shift-right: [w695] -> _
        shift-left: _ -> [w704]
        shift-right: ["pid reset left"] -> _
        shift-left: _ -> [w690]
        tunnel: [w696] -> _
        tunnel: w199 -> [w698]
        tunnel: w198 -> [w697]
        stop <- "pid reset left" stop-if-true
        # "*****\n\n(true is supposed\nto be 0)"
        n412 = call "Elapsed Time2"("Reset"=w690) -> ("Elapsed Time (s)"=w689:dbl, "Time has Elapsed"=w691:bool)  [unwired: 11 in, 6 out]
        "Elapsed Time (s) Left" <- w689
        n413 = local read "scale"() -> (w681:dbl)
        n414 = Not(x=w691) -> (.not. x?=w703:bool)
        ".not. x? 3" <- w703
        n415 = Greater?(x=w681, y=0.0) -> (0:w684:bool)
        n416 = Greater Or Equal?(x=w689, y=4.0) -> (x >= y?=w687:bool)
        n417 = case shown="False" w684 {
          tunnel: [w710 w711] -> w694
          frame False {
            n418 = local read "right setpoint"() -> (w710:dbl)
          }
          frame True {
            n419 = local read "left setpoint"() -> (w711:dbl)
          }
        }
        n420 = case shown="False" w687 {
          tunnel: [1.0 1.0] -> _
          frame False {
          }
          frame True {
          }
        }
        n421 = local read "big red button"() -> (w678:i16)
        n422 = Multiply(x=w694, y=w678) -> (x*y=w679:dbl)
        n423 = local read "stop motors"() -> (w699:dbl)
        n424 = local read "encoder stop switch"() -> (w692:dbl)
        n425 = Multiply(x=w681, y=w679) -> (x*y=w682:dbl)
        n426 = Multiply(x=w699, y=w682) -> (x*y=w693:dbl)
        n427 = Add(x=0.5, y=w682) -> (x+y=→"desired pwm left":dbl)
        n428 = Multiply(x=w693, y=w692) -> (x*y=w680:dbl)
        n429 = call-poly <vilib>:"PID.vi"("reinitialize? (F)"=w703, "output range"="output range left", "PID gains"="PID gains left", "process variable"=w704, "setpoint"=w680) -> ("dt out (s)"=→"dt out (s) left":dbl, "output"=w695:dbl)  [unwired: 5 in]
        n430 = Add(x=0.5, y=w695) -> (x+y=w685:dbl)
        "left wheels actual pwm" <- w685
        "left pwm" <- w685
        n431 = call <vilib>:"Set Duty Cycle and Frequency.vi"("Frequency [Hz]"=w696, "Duty Cycle"=w685, "PWM Ref In"=w697) -> ()  [unwired: 6 in, 2 out]
        n432 = call <vilib>:"Set Duty Cycle and Frequency.vi"("Frequency [Hz]"=w696, "Duty Cycle"=w685, "PWM Ref In"=w698) -> ()  [unwired: 6 in, 2 out]
        n433 = call <vilib>:"Set Duty Cycle and Frequency.vi"("Frequency [Hz]"=w696, "Duty Cycle"=w685, "PWM Ref In"=w708) -> ("PWM Ref Out"=w709:T9)  [unwired: 6 in, 1 out]
        "PID feedback Left" <- w704
      }
      n434 = while {
        tunnel: w206 -> [w814]
        stop <- FALSE stop-if-true
        # "left mid"
        n435 = xnode "Read/Write Control"("FPGA VI Reference In"=w814) -> ("ENC.A_a.CNTR"=→"ENC.A_a.CNTR":u32, "ENC.A_b.CNTR"=→"ENC.A_b.CNTR":u32, "ENC.A_c.CNTR"=→"ENC.A_c.CNTR":u32, "ENC.B_a.CNTR"=→"ENC.B_a.CNTR":u32, "ENC.B_b.CNTR"=→"ENC.B_b.CNTR":u32, "ENC.B_c.CNTR"=→"ENC.B_c.CNTR":u32)  [unwired: 1 in, 2 out]
        n436 = xnode "Read/Write Control"("FPGA VI Reference In"=w814) -> ("SYS.SELECTA"=→"SYS.SELECTA":u8)  [unwired: 1 in, 2 out]
        n437 = Wait (ms)(milliseconds to wait=u32 20) -> ()  [unwired: 1 out]
        n438 = case shown="True" "Encoder Reset" {
          tunnel: w814 -> [_ w825]
          frame False {
          }
          frame True {
            n439 = flat-sequence {
              tunnel: w825 -> [w830]
              tunnel: [w828] -> w827
              tunnel: w827 -> [w832]
              tunnel: [w832] -> w826
              tunnel: w826 -> [w835]
              tunnel: [w834] -> _
              frame #0 {
                w829 = u8 60 ("SYS.SELECTA")
                w831 = u8 3 ("ENC.B_c.CNFG")
                n440 = xnode "Read/Write Control"("FPGA VI Reference In"=w830, "ENC.A_a.CNFG"=w831, "ENC.A_b.CNFG"=w831, "ENC.A_c.CNFG"=w831, "ENC.B_a.CNFG"=w831, "ENC.B_b.CNFG"=w831, "ENC.B_c.CNFG"=w831, "SYS.SELECTA"=w829, "SYS.SELECTB"=w829) -> ("FPGA VI Reference Out"=w828:refnum<k20>)  [unwired: 1 in, 1 out]
              }
              frame #1 {
                n441 = Wait (ms)(milliseconds to wait=u32 10) -> ()  [unwired: 1 out]
              }
              frame #2 {
                w836 = u8 1 ("ENC.B_c.CNFG")
                n442 = xnode "Read/Write Control"("FPGA VI Reference In"=w835, "ENC.A_a.CNFG"=w836, "ENC.A_b.CNFG"=w836, "ENC.A_c.CNFG"=w836, "ENC.B_a.CNFG"=w836, "ENC.B_b.CNFG"=w836, "ENC.B_c.CNFG"=w836) -> ("FPGA VI Reference Out"=w834:refnum<k20>)  [unwired: 1 in, 1 out]
              }
            }
          }
        }
      }
      n443 = while {
        tunnel: w204 -> [w808]
        tunnel: [w809] -> _
        tunnel: [w797] -> _
        shift-right: [w796] -> _
        shift-left: _ -> [w804]
        shift-right: ["pid reset right"] -> _
        shift-left: _ -> [w790]
        tunnel: w202 -> [w797]
        tunnel: w201 -> [w799]
        tunnel: w200 -> [w798]
        stop <- "pid reset right" stop-if-true
        # "******"
        n444 = local read "scale"() -> (w783:dbl)
        n445 = Greater?(x=w783, y=0.0) -> (0:w781:bool)
        n446 = case shown="True" w781 {
          tunnel: [w810 w811] -> w780
          frame False {
            n447 = local read "left setpoint"() -> (w810:dbl)
          }
          frame True {
            n448 = local read "right setpoint"() -> (w811:dbl)
          }
        }
        n449 = call "Elapsed Time"("Reset"=w790) -> ("Elapsed Time (s)"=w789:dbl, "Time has Elapsed"=w787:bool)  [unwired: 11 in, 6 out]
        "Elapsed Time (s) Right" <- w789
        n450 = local read "big red button"() -> (w776:i16)
        n451 = local read "encoder stop switch"() -> (w793:dbl)
        n452 = Not(x=w787) -> (.not. x?=w803:bool)
        ".not. x? 2" <- w803
        n453 = Greater Or Equal?(x=w789, y=4.0) -> (x >= y?=w786:bool)
        n454 = Multiply(x=w776, y=w780) -> (x*y=w777:dbl)
        n455 = case shown="False" w786 {
          tunnel: [1.0 1.0] -> w791
          frame False {
          }
          frame True {
          }
        }
        n456 = Multiply(x=w783, y=w777) -> (x*y=w795:dbl)
        n457 = local read "stop motors"() -> (w784:dbl)
        n458 = Multiply(x=w795, y=w793) -> (x*y=w794:dbl)
        n459 = Add(x=0.5, y=w795) -> (x+y=→"desired pwm right":dbl)
        n460 = Multiply(x=w784, y=w794) -> (x*y=w785:dbl)
        n461 = Multiply(x=w785, y=w791) -> (x*y=w792:dbl)
        n462 = call-poly <vilib>:"PID.vi"("reinitialize? (F)"=w803, "output range"="output range right", "PID gains"="PID gains right", "process variable"=w804, "setpoint"=w792) -> ("dt out (s)"=→"dt out (s) right":dbl, "output"=w796:dbl)  [unwired: 5 in]
        n463 = Add(x=0.5, y=w796) -> (x+y=w778:dbl)
        "right wheels actual pwm" <- w778
        "right pwm" <- w778
        n464 = call <vilib>:"Set Duty Cycle and Frequency.vi"("Frequency [Hz]"=w797, "Duty Cycle"=w778, "PWM Ref In"=w799) -> ()  [unwired: 6 in, 2 out]
        n465 = call <vilib>:"Set Duty Cycle and Frequency.vi"("Frequency [Hz]"=w797, "Duty Cycle"=w778, "PWM Ref In"=w798) -> ()  [unwired: 6 in, 2 out]
        n466 = call <vilib>:"Set Duty Cycle and Frequency.vi"("Frequency [Hz]"=w797, "Duty Cycle"=w778, "PWM Ref In"=w808) -> ("PWM Ref Out"=w809:T9)  [unwired: 6 in, 1 out]
        "PID feedback Right" <- w804
      }
      n467 = while {
        stop <- FALSE stop-if-true
        # "(current-start)/(goal-start)"
        n468 = Not(x="motor killswitch") -> (.not. x?=w228:bool)
        n469 = local read "Encoder Reset"() -> (w230:bool)
        n470 = case shown="False" w230 {
          tunnel: [w240 w241] -> w229
          frame False {
            w240 = 1.0
            n471 = local write "reset x y 2"(w240) -> ()
          }
          frame True {
            w241 = 0.0
            n472 = local write "reset x y 2"(w241) -> ()
            "reset x y 2" <- w241
          }
        }
        "encoder stop switch" <- w229
        n473 = Boolean To (0,1)(Boolean=w228) -> (0, 1=→"big red button":i16)
        n474 = local read "x position 2"() -> (w224:dbl)
        n475 = local read "start x"() -> (w220:dbl)
        n476 = Subtract(x="x goal", y=w220) -> (x-y=w219:dbl)
        n477 = Subtract(x=w224, y=w220) -> (x-y=w223:dbl)
        n478 = Subtract(x=w220, y="x goal") -> (x-y=w222:dbl)
        n479 = Sign(1:w219) -> (0:w215:dbl)
        "scale" <- w215
        n480 = Divide(x=w223, y=w222) -> (x/y=w216:dbl)
        "percent to goal" <- w216
        n481 = Greater?(x=w216, y=0.75) -> (0:w217:bool)
        n482 = case shown="True" w217 {
          tunnel: w215 -> [w231 w233]
          tunnel: w216 -> [_ w234]
          frame False {
            n483 = Multiply(x=1.0, y=w231) -> ()  [unwired: 1 out]
          }
          frame True {
            n484 = Greater?(x=w234, y=1.001) -> (0:w235:bool)
            n485 = case shown="True" w235 {
              tunnel: w233 -> [w238 _]
              frame False {
                n486 = Multiply(x=w238, y=1.0) -> ()  [unwired: 1 out]
              }
              frame True {
                "goal reached" <- TRUE
              }
            }
          }
        }
      }
      n487 = while {
        shift-right: [w724] -> _
        shift-left: _ -> [w762]
        shift-right: [w721] -> _
        shift-left: _ -> [w761]
        shift-right: [w723] -> _
        shift-left: _ -> [w736]
        shift-right: [w722] -> _
        shift-left: _ -> [w735]
        stop <- FALSE stop-if-true
        w757 = 28.0  # width wheel to wheel
        w758 = 4.0  # wheel radius
        n488 = local read "reset x y 2"() -> (w720:dbl)
        n489 = call "Wait3"("Count(mSec)"=u32 20) -> ("Tick Count(mSec)"=→"Tick Count(mSec) 2":u32)
        n490 = Multiply(x=w720, y=w735) -> (x*y=w726:dbl)
        n491 = Multiply(x=w720, y=w762) -> (x*y=w728:dbl)
        n492 = Multiply(x=w720, y=w761) -> (x*y=w725:dbl)
        n493 = Multiply(x=w720, y=w736) -> (x*y=w727:dbl)
        n494 = local read "ENC.A_b.CNTR"() -> (w769:i32)
        n495 = local read "ENC.A_c.CNTR"() -> (w768:i32)
        n496 = local read "ENC.B_a.CNTR"() -> (w767:i32)
        n497 = local read "ENC.B_b.CNTR"() -> (w766:i32)
        n498 = local read "ENC.A_a.CNTR"() -> (w770:i32)
        n499 = local read "ENC.B_c.CNTR"() -> (w765:i32)
        n500 = Compound Arithmetic op=ADD(w770, w769, w768) -> (w774:i32)
        n501 = Compound Arithmetic op=ADD(w767, w766, w765) -> (w773:i32)
        n502 = Divide(x=w774, y=2) -> (x/y=w763:dbl)
        "avg ENC.A" <- w763
        n503 = Divide(x=w773, y=3) -> (x/y=w760:dbl)
        "avg ENC.B" <- w760
        n504 = Subtract(x=w763, y=w728) -> (x-y=w751:dbl)
        n505 = Subtract(x=w760, y=w725) -> (x-y=w750:dbl)
        n506 = Add(x=w751, y=w750) -> (x+y=w755:dbl)
        n507 = Divide(x=w758, y=w757) -> (x/y=w753:dbl)
        n508 = Square(x=w751) -> (x^2=w748:dbl)
        n509 = Square(x=w750) -> (x^2=w749:dbl)
        n510 = Subtract(x=w751, y=w750) -> (x-y=w754:dbl)
        n511 = Divide(x=w758, y=2.0) -> (x/y=w756:dbl)
        n512 = Add(x=w748, y=w749) -> (x+y=w747:dbl)
        n513 = Multiply(x=w754, y=w753) -> (x*y=→"psi dot 2":dbl)
        n514 = Multiply(x=w755, y=w756) -> (x*y=w744:dbl)
        n515 = Inverse Tangent(1:w754) -> (0:w752:dbl)
        n516 = Cosine(x=w752) -> (cos(x)=w745:dbl)
        n517 = Sine(x=w752) -> (sin(x)=w746:dbl)
        n518 = local read "reset x y 2"() -> (w718:dbl)
        n519 = Square Root(x=w747) -> (sqrt(x)=w741:dbl)
        n520 = Multiply(x=w744, y=w745) -> (x*y=w742:dbl)
        "x dot 2" <- w742
        n521 = Multiply(x=w744, y=w746) -> (x*y=w743:dbl)
        "y dot 2" <- w743
        n522 = Multiply(x=w763, y=w718) -> (x*y=w724:dbl)
        n523 = Multiply(x=w760, y=w718) -> (x*y=w721:dbl)
        n524 = Multiply(x=w741, y=w718) -> (x*y=w719:dbl)
        "distance traveled 2" <- w719
        n525 = Multiply(x=w719, y=w742) -> (x*y=w740:dbl)
        "x traveled 2" <- w740
        n526 = Multiply(x=w719, y=w743) -> (x*y=w739:dbl)
        "y traveled 2" <- w739
        n527 = Add(x=w726, y=w740) -> (x+y=w738:dbl)
        n528 = Add(x=w727, y=w739) -> (x+y=w730:dbl)
        n529 = Multiply(x=w738, y=w718) -> (x*y=w722:dbl)
        n530 = Multiply(x=w718, y=w730) -> (x*y=w723:dbl)
        n531 = Divide(x=w738, y=9600.0) -> (x/y=w733:dbl)
        n532 = Divide(x=w730, y=9600.0) -> (x/y=w734:dbl)
        n533 = local read "start x"() -> (w731:dbl)
        n534 = local read "start y"() -> (w732:dbl)
        n535 = Add(x=w733, y=w731) -> (x+y=→"x position 2":dbl)
        n536 = Add(x=w734, y=w732) -> (x+y=→"y position 2":dbl)
      }
      n537 = while {
        shift-right: [w855] -> _
        shift-left: _ -> [w854]
        shift-right: [w852] -> _
        shift-left: w207 -> [w851]
        tunnel: w205 -> [w862]
        stop <- FALSE stop-if-true
        n538 = xnode "Read/Write Control"("FPGA VI Reference In"=w862) -> ("ENC.A_a.CNTR"=w861:u32, "ENC.A_b.CNTR"=w860:u32, "ENC.A_c.CNTR"=w859:u32, "ENC.B_a.CNTR"=w858:u32, "ENC.B_b.CNTR"=w857:u32, "ENC.B_c.CNTR"=w856:u32)  [unwired: 1 in, 2 out]
        n539 = call "Wait"("Count(mSec)"=u32 20) -> ()  [unwired: 1 out]
        n540 = Build Array(w861, w860, w859, w858, w857, w856) -> (w855:u32[])
        n541 = Subtract(x=w855, y=w854) -> (x-y=w853:u32[])
        n542 = call "Tick Count2"() -> ("Tick Count(uSec)"=w852:u32)
        n543 = Index Array(array=w853) -> (element #1=w850:u32, element #2=w849:u32, element #3=w848:u32, element #4=w847:u32, element #5=w846:u32, element #6=w845:u32)  [unwired: 6 in]
        n544 = Subtract(x=w852, y=w851) -> (x-y=w844:u32)
        n545 = call "Encoder-Velocity_Conversion (SubVI).vi"("delta  Encoder Count"=w850, "dt (uSec)"=w844) -> ("Rotational Velocity (RPS)"=w840:dbl)  [unwired: 7 in, 2 out]
        "LR Rot Velocity (rot/s)" <- w840
        n546 = call "Encoder-Velocity_Conversion (SubVI).vi"("delta  Encoder Count"=w845, "dt (uSec)"=w844) -> ("Rotational Velocity (RPS)"=w842:dbl)  [unwired: 7 in, 2 out]
        "RF Linear Velocity (rot/s)" <- w842
        n547 = call "Encoder-Velocity_Conversion (SubVI).vi"("delta  Encoder Count"=w849, "dt (uSec)"=w844) -> ("Rotational Velocity (RPS)"=w839:dbl)  [unwired: 7 in, 2 out]
        "LM Rot Velocity (rot/s)" <- w839
        n548 = call "Encoder-Velocity_Conversion (SubVI).vi"("delta  Encoder Count"=w848, "dt (uSec)"=w844) -> ("Rotational Velocity (RPS)"=w838:dbl)  [unwired: 7 in, 2 out]
        "LF Rot Velocity (rot/s)" <- w838
        n549 = call "Encoder-Velocity_Conversion (SubVI).vi"("delta  Encoder Count"=w847, "dt (uSec)"=w844) -> ("Rotational Velocity (RPS)"=w837:dbl)  [unwired: 7 in, 2 out]
        "RR Rot Velocity (rot/s)" <- w837
        n550 = call "Encoder-Velocity_Conversion (SubVI).vi"("delta  Encoder Count"=w846, "dt (uSec)"=w844) -> ("Rotational Velocity (RPS)"=w841:dbl)  [unwired: 7 in, 2 out]
        "RM Linear Velocity (rot/s)" <- w841
        n551 = Bundle("Rotational Velocity (RPS)"=w840, "Rotational Velocity (RPS)"=w839, "Rotational Velocity (RPS)"=w838, "Rotational Velocity (RPS)"=w837, "Rotational Velocity (RPS)"=w841, "Rotational Velocity (RPS)"=w842) -> (→"Current Rot Velocity (rot/s)":T6)  [unwired: 1 in]
      }
    }
  }
